vi "CPP-Multiplot.vi"(0 "PlotArray":cluster{dbl[], dbl[]}[](array[cluster]), 1 "Job Directory":path) -> (2 "Saved Automatically?":bool, 3 "gnuplotScript":string, 4 "Plot data file":path)   [LabVIEW 2017]
uses:
  gnuplotScriptComponents/plotstyle.ctl
  gnuplotScriptComponents/graphPeripherals.ctl
  gnuplotScriptComponents/minAndMax.ctl
  gnuplotScriptComponents/AutoManualNumber.ctl
  gnuplotScriptComponents/ticsAndGrids.ctl
  gnuplotScriptComponents/tics.ctl
  gnuplotScriptComponents/grids.ctl
  gnuplotScriptComponents/legendProperties.ctl
  gnuplotScriptComponents/legendAppearance.ctl
  gnuplotScriptComponents/alignment.ctl
  gnuplotScriptComponents/at.ctl
  gnuplotScriptComponents/margins.ctl
  gnuplotScriptComponents/source.ctl
  gnuplotScriptComponents/Master_Legend.ctl
  gnuplotScriptComponents/MasterPeripherals.ctl
  Error bar Type.ctl
  gnuplotScriptComponents/axisName.ctl
  Results_plotter_Global.vi
panel:
  out "Multi_Plot":bool
  in  "OpenLogfile?":bool
  in  "Show Script Editor?":bool
  in  "Tab Control":T1(tab)=enum."Appearance"
  in  "Each Graph contains:":T2=enum."Series"
  in  "Rows from:":T2=enum."Until done"
  in  "Columns from:":T2=enum."Yellow Filter"
  in  "Margins":T3={"Top"=2.0, "Bottom"=2.0, "Left"=2.0, "Right"=2.0}
  in  "Height (in)":dbl=7.0 min=0.5 step=0.5 format="%.1f"
  in  "Width (in)":dbl=10.0 min=0.5 step=0.5 format="%.1f"
  in  "nRows":u8=3 min=1
  in  "nCols":u8=3 min=1
  in  "ScaleAdjust":dbl=0.9 min=0.1 max=2.0 step=0.1
  in  "PlotTitlesNeed $$?":bool=TRUE
  in  "Show Channels with range of Values?":bool
  in  "ManualPlotTitles":string[](array[string])
  out "AutoPlotTitles":string[](array[string])
  in  "Individual Plot Titles":bool=TRUE
  in  "Page Title Pre Block":string
  in  "Page Title Post Block":string
  in  "Values to include in Page Title":i32[](listbox)
  in  "Plot Title Offset (characters)":cluster{"horizontal":dbl, "vertical":dbl}
  out "Final Title":string
  in  "PlotNamesNeed $$?":bool=TRUE
  in  "Plot Legends Manual":string[](array[string])
  in  "Plotstyles":T4[](array[typedef])=[{"Style"="linespoints", "Color"=16711680, "PointType"=1, "PointSize"=1.0, "LineWidth"=1.0, "LineType"=1}, {"Style"="linespoints", "Color"=16860, "PointType"=2, "PointSize"=1.0, "LineWidth"=1.0, "LineType"=1}, {"Style"="linespoints", "Color"=51228, "PointType"=3, "PointSize"=1.0, "LineWidth"=1.0, "LineType"=1}, {"Style"="linespoints", "Color"=0, "PointType"=4, "PointSize"=1.0, "LineWidth"=1.0, "LineType"=1}, {"Style"="linespoints", "Color"=9567230, "PointType"=5, "PointSize"=1.0, "LineWidth"=1.0, "LineType"=1}, {"Style"="linespoints", "Color"=12369084, "PointType"=6, "PointSize"=1.0, "LineWidth"=1.0, "LineType"=1}, {"Style"="linespoints", "Color"=15667967, "PointType"=7, "PointSize"=1.0, "LineWidth"=1.0, "LineType"=1}, {"Style"="linespoints", "Color"=15400704, "PointType"=8, "PointSize"=1.0, "LineWidth"=1.0, "LineType"=1}, {"Style"="linespoints", "Color"=128, "PointType"=9, "PointSize"=1.0, "LineWidth"=1.0, "LineType"=1}, {"Style"="linespoints", "Color"=8404992, "PointType"=10, "PointSize"=1.0, "LineWidth"=1.0, "LineType"=1}, {"Style"="linespoints", "Color"=6737151, "PointType"=11, "PointSize"=1.0, "LineWidth"=1.0, "LineType"=1}, {"Style"="linespoints", "Color"=8388672, "PointType"=12, "PointSize"=1.0, "LineWidth"=1.0, "LineType"=1}, {"Style"="linespoints", "Color"=16740303, "PointType"=13, "PointSize"=1.0, "LineWidth"=1.0, "LineType"=1}, {"Style"="linespoints", "Color"=16764006, "PointType"=14, "PointSize"=1.0, "LineWidth"=1.0, "LineType"=1}, {"Style"="linespoints", "Color"=8421376, "PointType"=15, "PointSize"=1.0, "LineWidth"=1.0, "LineType"=1}, {"Style"="linespoints", "Color"=65408, "PointType"=16, "PointSize"=1.0, "LineWidth"=1.0, "LineType"=1}] caption="Style                              Colour  PointType    PointSize     Linewidth      Linestyle" {"LineType" min=1 max=6 step=1; "LineWidth" min=1 max=6 step=1; "PointSize" min=0 step=0.1}
  out "Plot Legends Auto":string[](array[string])
  out "No of Series supplied":i32
  out "No of Graph Slots Available":i32
  in  "Plot Legends":bool=TRUE
  in  "Error Bar Type":T5
  in  "X axis label":enum32{"Autolabel", "Manual Label"}(tab)
  out "X or theta label":string
  in  "X or theta label Manual":string
  in  "LegendProperties":T6={"Appearance"={"layout"="", "text-sample order"="", "key order"="", "surroundingBox"="", "MaxRows"=0, "MaxCols"=0, "WidthAdjust"=0.0}, "Alignment"={"Horizontal"="", "Vertical"=""}, "Location"="auto", "\"At\" location"={"XcoordSys"="", "YcoordSys"="", "Xvalue"=0.0, "Yvalue"=0.0}}
  in  "Y/R tics And Grids":T10={"tics"={"ticMin"=0.0, "ticStep"=5.0, "ticMax"=0.0, "minorDivsPerMajor"=2, "ticSpacing"=enum."Approx n Tics (rounded)", "ticPosition"=enum."Inside, no mirror"}, "Grids"={"Gridlines"=enum."No grids", "Zeroaxis"=enum."No zero axis"}, "Mapping"=enum."Lin"}
  in  "X/Theta tics And Grids":T10={"tics"={"ticMin"=0.0, "ticStep"=5.0, "ticMax"=0.0, "minorDivsPerMajor"=2, "ticSpacing"=enum."Approx n Tics (rounded)", "ticPosition"=enum."Inside, no mirror"}, "Grids"={"Gridlines"=enum."Major grid", "Zeroaxis"=enum."No zero axis"}, "Mapping"=enum."Lin"}
  in  "PlotType":enum32{"XY", "Polar", "Time"}(tab)
  in  "yAxisBounds":T13={"Min"={"Auto"=TRUE, "Value"=0.0}, "Max"={"Auto"=TRUE, "Value"=0.0}}
  in  "Additional XYgnuplot":string
  in  "xAxisBounds":T13={"Min"={"Auto"=TRUE, "Value"=0.0}, "Max"={"Auto"=TRUE, "Value"=0.0}}
  in  "Set bounds using XY Plot \non Results file plotter":bool
  in  "Angle Units":bool=TRUE
  in  "AngleMode":string(combo)="Compass"
  in  "wrapGapsUpTo:":dbl=30.0 step=0.1
  in  "Additional Polar gnuplot":string
  in  "rAxisBounds":T13={"Min"={"Auto"=FALSE, "Value"=0.0}, "Max"={"Auto"=FALSE, "Value"=1.5}}
  out "Time format?":bool
  in  "Time/Date Format":string(combo)="%I:%M %p\\n%d-%b-%y"
  in  "Select Time Zone":u32(ring)=142 items=["Abbreviation (Time Zone Name)", "A (Alpha Time Zone)", "ACDT (Australian Central Daylight Time  CDT ‚Äì Central Daylight Time CDST ‚Äì Central Daylight Savings Time)", "ACST (Australian Central Standard Time  CST ‚Äì Central Standard Time)", "ACT (Acre Time)", "ACT (Australian Central Time)", "ACWST (Australian Central Western Standard Time)", "ADT (Arabia Daylight Time  AST ‚Äì Arabia Summer Time)", "ADT (Atlantic Daylight Time  ADST ‚Äì Atlantic Daylight Saving Time AST ‚Äì Atlantic Summer Time  HAA ‚Äì Heure Avancv©e de l'Atlantique (French))", "AEDT (Australian Eastern Daylight Time  EDT ‚Äì Eastern Daylight Time EDST ‚Äì Eastern Daylight Saving Time)", "AEST (Australian Eastern Standard Time  EST ‚Äì Eastern Standard Time AET ‚Äì Australian Eastern Time)", "AET (Australian Eastern Time)", "AFT (Afghanistan Time)", "AKDT (Alaska Daylight Time  ADST ‚Äì Alaska Daylight Saving Time)", "AKST (Alaska Standard Time  AT ‚Äì Alaska Time)", "ALMT (Alma-Ata Time)", "AMST (Amazon Summer Time)", "AMST (Armenia Summer Time  AMDT ‚Äì Armenia Daylight Time)", "AMT (Amazon Time)", "AMT (Armenia Time)", "ANAST (Anadyr Summer Time)", "ANAT (Anadyr Time)", "AQTT (Aqtobe Time)", "ART (Argentina Time)", "AST (Arabia Standard Time  AST ‚Äì Arabic Standard Time AST ‚Äì Al Manamah Standard Time)", "AST (Atlantic Standard Time  AT ‚Äì Atlantic Time  AST ‚Äì Tiempo Estv°ndar del Atlv°ntico (Spanish) HNA ‚Äì Heure Normale de l'Atlantique (French))", "AT (Atlantic Time)", "AWDT (Australian Western Daylight Time  WDT ‚Äì Western Daylight Time WST ‚Äì Western Summer Time)", "AWST (Australian Western Standard Time  WST ‚Äì Western Standard Time WAT ‚Äì Western Australia Time)", "AZOST (Azores Summer Time  AZODT ‚Äì Azores Daylight Time)", "AZOT (Azores Time  AZOST ‚Äì Azores Standard Time)", "AZST (Azerbaijan Summer Time)", "AZT (Azerbaijan Time)", "AoE (Anywhere on Earth)", "B (Bravo Time Zone)", "BNT (Brunei Darussalam Time  BDT ‚Äì Brunei Time)", "BOT (Bolivia Time)", "BRST (Brasv?lia Summer Time  BST ‚Äì Brazil Summer Time BST ‚Äì Brazilian Summer Time)", "BRT (Brasv?lia Time  BT ‚Äì Brazil Time BT ‚Äì Brazilian Time)", "BST (Bangladesh Standard Time)", "BST (Bougainville Standard Time)", "BST (British Summer Time  BDT ‚Äì British Daylight Time BDST ‚Äì British Daylight Saving Time)", "BTT (Bhutan Time)", "C (Charlie Time Zone)", "CAST (Casey Time)", "CAT (Central Africa Time)", "CCT (Cocos Islands Time)", "CDT (Central Daylight Time  CDST ‚Äì Central Daylight Saving Time NACDT ‚Äì North American Central Daylight Time  HAC ‚Äì Heure Avancv©e du Centre (French))", "CDT (Cuba Daylight Time)", "CEST (Central European Summer Time  CEDT ‚Äì Central European Daylight Time ECST ‚Äì European Central Summer Time  MESZ ‚Äì Mitteleuropv§ische Sommerzeit (German))", "CET (Central European Time  ECT ‚Äì European Central Time CET ‚Äì Central Europe Time  MEZ ‚Äì Mitteleuropv§ische Zeit (German))", "CHADT (Chatham Island Daylight Time  CDT ‚Äì Chatham Daylight Time)", "CHAST (Chatham Island Standard Time)", "CHOST (Choibalsan Summer Time  CHODT ‚Äì Choibalsan Daylight Time CHODST ‚Äì Choibalsan Daylight Saving Time)", "CHOST (Choibalsan Summer Time)", "CHOT (Choibalsan Time)", "CHUT (Chuuk Time)", "CIDST (Cayman Islands Daylight Saving Time)", "CIST (Cayman Islands Standard Time  CIT ‚Äì Cayman Islands Time)", "CKT (Cook Island Time)", "CLST (Chile Summer Time  CLDT ‚Äì Chile Daylight Time)", "CLT (Chile Standard Time  CT ‚Äì Chile Time CLST ‚Äì Chile Standard Time)", "COT (Colombia Time)", "CST (Central Standard Time  CT ‚Äì Central Time NACST ‚Äì North American Central Standard Time  CST ‚Äì Tiempo Central Estv°ndar (Spanish) HNC ‚Äì Heure Normale du Centre (French))", "CST (China Standard Time)", "CST (Cuba Standard Time)", "CT (Central Time)", "CVT (Cape Verde Time)", "CXT (Christmas Island Time)", "ChST (Chamorro Standard Time  GST ‚Äì Guam Standard Time)", "D (Delta Time Zone)", "DAVT (Davis Time)", "DDUT (Dumont-d'Urville Time)", "E (Echo Time Zone)", "EASST (Easter Island Summer Time  EADT ‚Äì Easter Island Daylight Time)", "EAST (Easter Island Standard Time)", "EAT (Eastern Africa Time  EAT ‚Äì East Africa Time)", "ECT (Ecuador Time)", "EDT (Eastern Daylight Time  EDST ‚Äì Eastern Daylight Savings Time NAEDT ‚Äì North American Eastern Daylight Time  HAE ‚Äì Heure Avancv©e de l'Est (French) EDT ‚Äì Tiempo de verano del Este (Spanish))", "EEST (Eastern European Summer Time  EEDT ‚Äì Eastern European Daylight Time  OESZ ‚Äì Osteuropv§ische Sommerzeit (German))", "EET (Eastern European Time  OEZ ‚Äì Osteuropv§ische Zeit (German))", "EGST (Eastern Greenland Summer Time  EGST ‚Äì East Greenland Summer Time)", "EGT (East Greenland Time  EGT ‚Äì Eastern Greenland Time)", "EST (Eastern Standard Time  ET ‚Äì Eastern Time  NAEST ‚Äì North American Eastern Standard Time  ET ‚Äì Tiempo del Este (Spanish) HNE ‚Äì Heure Normale de l'Est (French))", "ET (Eastern Time)", "F (Foxtrot Time Zone)", "FET (Further-Eastern European Time)", "FJST (Fiji Summer Time  FJDT ‚Äì Fiji Daylight Time)", "FJT (Fiji Time)", "FKST (Falkland Islands Summer Time  FKDT ‚Äì Falkland Island Daylight Time)", "FKT (Falkland Island Time  FKST ‚Äì Falkland Island Standard Time)", "FNT (Fernando de Noronha Time)", "G (Golf Time Zone)", "GALT (Galapagos Time)", "GAMT (Gambier Time  GAMT ‚Äì Gambier Islands Time)", "GET (Georgia Standard Time)", "GFT (French Guiana Time)", "GILT (Gilbert Island Time)", "GMT (Greenwich Mean Time  \"‚Äì Coordinated Universal Time GT ‚Äì Greenwich Time)", "GST (Gulf Standard Time)", "GST (South Georgia Time)", "GYT (Guyana Time)", "H (Hotel Time Zone)", "HADT (Hawaii-Aleutian Daylight Time  HDT ‚Äì Hawaii Daylight Time)", "HAST (Hawaii-Aleutian Standard Time  HST ‚Äì Hawaii Standard Time)", "HKT (Hong Kong Time)", "HOVST (Hovd Summer Time  HOVDT ‚Äì Hovd Daylight Time HOVDST ‚Äì Hovd Daylight Saving Time)", "HOVST (Hovd Summer Time)", "HOVT (Hovd Time)", "I (India Time Zone)", "ICT (Indochina Time)", "IDT (Israel Daylight Time)", "IOT (Indian Chagos Time)", "IRDT (Iran Daylight Time  IRST ‚Äì Iran Summer Time IDT ‚Äì Iran Daylight Time)", "IRKST (Irkutsk Summer Time)", "IRKT (Irkutsk Time)", "IRST (Iran Standard Time  IT ‚Äì Iran Time)", "IST (India Standard Time  IT ‚Äì India Time IST ‚Äì Indian Standard Time)", "IST (Irish Standard Time  IST ‚Äì Irish Summer Time)", "IST (Israel Standard Time)", "JST (Japan Standard Time)", "K (Kilo Time Zone)", "KGT (Kyrgyzstan Time)", "KOST (Kosrae Time)", "KRAST (Krasnoyarsk Summer Time)", "KRAT (Krasnoyarsk Time)", "KST (Korea Standard Time  KST ‚Äì Korean Standard Time KT ‚Äì Korea Time)", "KUYT (Kuybyshev Time  SAMST ‚Äì Samara Summer Time)", "L (Lima Time Zone)", "LHDT (Lord Howe Daylight Time)", "LHST (Lord Howe Standard Time)", "LINT (Line Islands Time)", "M (Mike Time Zone)", "MAGST (Magadan Summer Time  MAGST ‚Äì Magadan Island Summer Time)", "MAGT (Magadan Time  MAGT ‚Äì Magadan Island Time)", "MART (Marquesas Time)", "MAWT (Mawson Time)", "MDT (Mountain Daylight Time  MDST ‚Äì Mountain Daylight Saving Time NAMDT ‚Äì North American Mountain Daylight Time  HAR ‚Äì Heure Avancv©e des Rocheuses (French))", "MHT (Marshall Islands Time)", "MMT (Myanmar Time)", "MSD (Moscow Daylight Time  Moscow Summer Time)", "MSK (Moscow Standard Time  MCK ‚Äì Moscow Time)", "MST (Mountain Standard Time  MT ‚Äì Mountain Time NAMST ‚Äì North American Mountain Standard Time  HNR ‚Äì Heure Normale des Rocheuses (French))", "MT (Mountain Time)", "MUT (Mauritius Time)", "MVT (Maldives Time)", "MYT (Malaysia Time  MST ‚Äì Malaysian Standard Time)", "N (November Time Zone)", "NCT (New Caledonia Time)", "NDT (Newfoundland Daylight Time  HAT ‚Äì Heure Avancv©e de Terre-Neuve (French))", "NFT (Norfolk Time  NFT ‚Äì Norfolk Island Time)", "NOVST (Novosibirsk Summer Time  OMSST ‚Äì Omsk Summer Time)", "NOVT (Novosibirsk Time  OMST ‚Äì Omsk Standard Time)", "NPT (Nepal Time)", "NRT (Nauru Time)", "NST (Newfoundland Standard Time  HNT ‚Äì Heure Normale de Terre-Neuve (French))", "NUT (Niue Time)", "NZDT (New Zealand Daylight Time)", "NZST (New Zealand Standard Time)", "O (Oscar Time Zone)", "OMSST (Omsk Summer Time  NOVST ‚Äì Novosibirsk Summer Time)", "OMST (Omsk Standard Time  OMST ‚Äì Omsk Time NOVT ‚Äì Novosibirsk Time)", "ORAT (Oral Time)", "P (Papa Time Zone)", "PDT (Pacific Daylight Time  PDST ‚Äì Pacific Daylight Saving Time NAPDT ‚Äì North American Pacific Daylight Time  HAP ‚Äì Heure Avancv©e du Pacifique (French))", "PET (Peru Time)", "PETST (Kamchatka Summer Time)", "PETT (Kamchatka Time  PETT ‚Äì Petropavlovsk-Kamchatski Time)", "PGT (Papua New Guinea Time)", "PHOT (Phoenix Island Time)", "PHT (Philippine Time  PST ‚Äì Philippine Standard Time)", "PKT (Pakistan Standard Time  PKT ‚Äì Pakistan Time)", "PMDT (Pierre & Miquelon Daylight Time)", "PMST (Pierre & Miquelon Standard Time)", "PONT (Pohnpei Standard Time)", "PST (Pacific Standard Time  PT ‚Äì Pacific Time NAPST ‚Äì North American Pacific Standard Time  PT ‚Äì Tiempo del Pacv?fico (Spanish) HNP ‚Äì Heure Normale du Pacifique (French))", "PST (Pitcairn Standard Time)", "PT (Pacific Time)", "PWT (Palau Time)", "PYST (Paraguay Summer Time)", "PYT (Paraguay Time)", "PYT (Pyongyang Time  PYST ‚Äì Pyongyang Standard Time)", "PYT (Pyongyang Time)", "Q (Quebec Time Zone)", "QYZT (Qyzylorda Time)", "R (Romeo Time Zone)", "RET (Reunion Time)", "ROTT (Rothera Time)", "S (Sierra Time Zone)", "SAKT (Sakhalin Time)", "SAMT (Samara Time  SAMT ‚Äì Samara Standard Time)", "SAST (South Africa Standard Time  SAST ‚Äì South African Standard Time)", "SBT (Solomon Islands Time  SBT ‚Äì Solomon Island Time)", "SCT (Seychelles Time)", "SGT (Singapore Time  SST ‚Äì Singapore Standard Time)", "SRET (Srednekolymsk Time)", "SRT (Suriname Time)", "SST (Samoa Standard Time)", "SYOT (Syowa Time)", "T (Tango Time Zone)", "TAHT (Tahiti Time)", "TFT (French Southern and Antarctic Time  KIT ‚Äì Kerguelen (Islands) Time)", "TJT (Tajikistan Time)", "TKT (Tokelau Time)", "TLT (East Timor Time)", "TMT (Turkmenistan Time)", "TOT (Tonga Time)", "TVT (Tuvalu Time)", "U (Uniform Time Zone)", "ULAST (Ulaanbaatar Summer Time  ULAST ‚Äì Ulan Bator Summer Time)", "ULAST (Ulaanbaatar Summer Time)", "ULAT (Ulaanbaatar Time  ULAT ‚Äì Ulan Bator Time)", "ULAT (Ulaanbaatar Time)", "UTC (Coordinated Universal Time)", "UYST (Uruguay Summer Time)", "UYT (Uruguay Time)", "UZT (Uzbekistan Time)", "V (Victor Time Zone)", "VET (Venezuelan Standard Time  HLV ‚Äì Hora Legal de Venezuela (Spanish))", "VLAST (Vladivostok Summer Time)", "VLAT (Vladivostok Time)", "VOST (Vostok Time)", "VUT (Vanuatu Time  EFATE ‚Äì Efate Time)", "W (Whiskey Time Zone)", "WAKT (Wake Time)", "WARST (Western Argentine Summer Time)", "WAST (West Africa Summer Time)", "WAT (West Africa Time)", "WEST (Western European Summer Time  WEDT ‚Äì Western European Daylight Time  WESZ ‚Äì Westeuropv§ische Sommerzeit (German))", "WET (Western European Time  GMT ‚Äì Greenwich Mean Time  WEZ ‚Äì Westeuropv§ische Zeit (German))", "WFT (Wallis and Futuna Time)", "WGST (Western Greenland Summer Time  WGST ‚Äì West Greenland Summer Time)", "WGT (West Greenland Time  WGT ‚Äì Western Greenland Time)", "WIB (Western Indonesian Time  WIB ‚Äì Waktu Indonesia Barat)", "WIT (Eastern Indonesian Time  WIT ‚Äì Waktu Indonesia Timur)", "WITA (Central Indonesian Time  WITA ‚Äì Waktu Indonesia Tengah)", "WST (West Samoa Time  ST ‚Äì Samoa Time)", "WST (Western Sahara Summer Time)", "WT (Western Sahara Standard Time  WT ‚Äì Western Sahara Time)", "X (X-ray Time Zone)", "Y (Yankee Time Zone)", "YAKST (Yakutsk Summer Time)", "YAKT (Yakutsk Time)", "YAPT (Yap Time)", "YEKST (Yekaterinburg Summer Time)", "YEKT (Yekaterinburg Time)", "Z (Zulu Time Zone)"]
  out "Time Format String":string="%I:%M %p\\n%d-%b-%y"
  out "Formatted date/time string":string="05:00 PM\\n21-Jan-16"
  out "TZ Shift (hrs)":string="UTC-7.00"
  in  "Y axis label":enum32{"Autolabel", "Manual Label"}(tab)
  out "Y or R label":string
  in  "Y or R label Manual 2":string
  in  "PeripheralsMasterControl":T15=enum."Edges Only"
  in  "Legend Options":T16=enum."Single Legend Below table"
  in  "GraphPeripherals":T17[][](array[typedef])
  out "PlotCommand":string
  in  "Filename Max length":i32=55
  out "File Path Control":path
  out "AuditTrail":string[](array[string])
  out "Desired Legends":string[][](array[string])
  out "original name had conflict":bool
  out "crossplatform problem":bool
  # "Rows/ Columns/ Series from: controls not wired- just a thought for explicit control of what goes where...?"
  # "Overall Page Title"
  # "There are as many graphs as there are titles (from Selector 2)...."
  # "Plot Styles"
  # "Each graph contains plots from Selector 1..."
  # "X/theta"
  # "Y/r"
  # "Shows the numbered line colours and point styles available- well it would, if it didn't disappear every time I update from the repository..!"
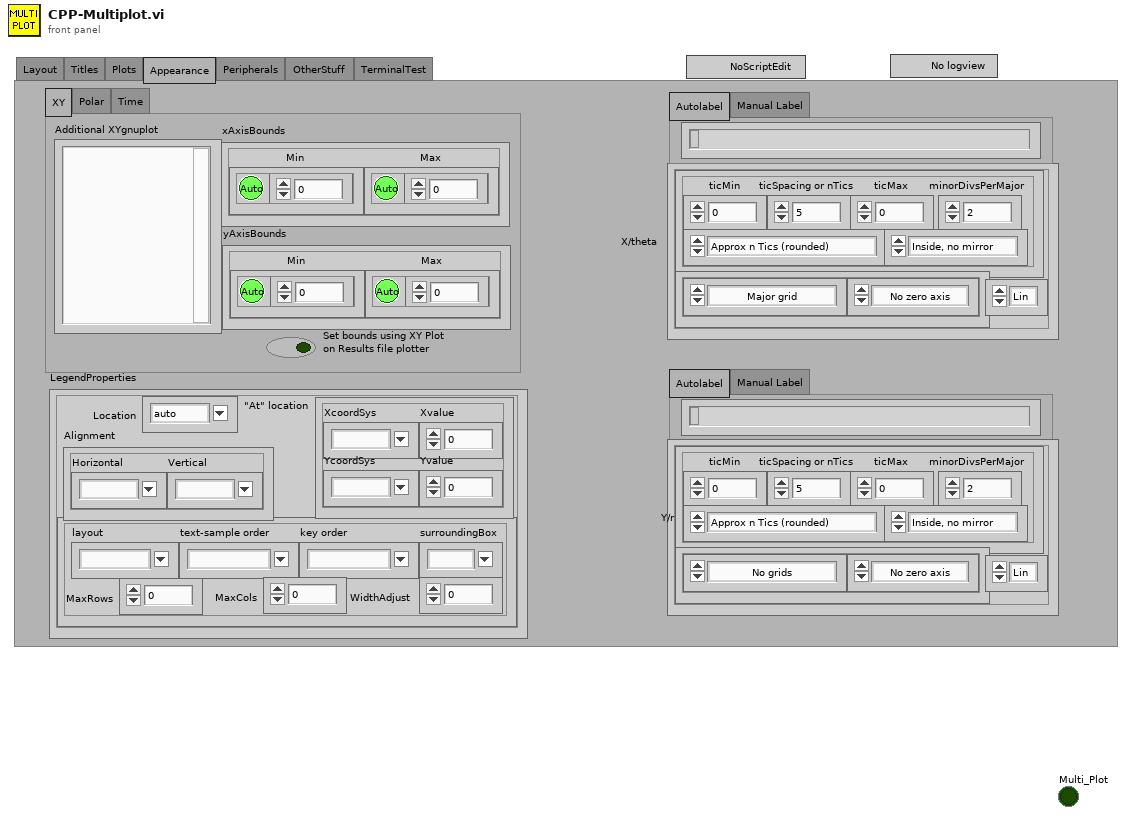
[diagram p1: front panel]
types:
  T1 = enum32{"Layout", "Titles", "Plots", "Appearance", "Peripherals", "OtherStuff ", "TerminalTest"}
  T2 = typedef "source.ctl" = enum16{"Specified:", "Yellow Filter", "Red Filter", "Until done", "Series"}
  T3 = typedef "margins.ctl" = cluster{"Top":dbl, "Bottom":dbl, "Left":dbl, "Right":dbl}
  T4 = typedef "plotstyle.ctl" = cluster{"Style":string, "Color":u32, "PointType":i32, "PointSize":sgl, "LineWidth":sgl, "LineType":u8}
  T5 = typedef "Error bar Type.ctl" = enum16{"Standard Error", "Separate upper and lower"}
  T6 = typedef "legendProperties.ctl" = cluster{"Appearance":T7, "Alignment":T8, "Location":string, "\"At\" location":T9}
  T7 = typedef "legendAppearance.ctl" = cluster{"layout":string, "text-sample order":string, "key order":string, "surroundingBox":string, "MaxRows":u32, "MaxCols":u32, "WidthAdjust":dbl}
  T8 = typedef "alignment.ctl" = cluster{"Horizontal":string, "Vertical":string}
  T9 = typedef "at.ctl" = cluster{"XcoordSys":string, "YcoordSys":string, "Xvalue":dbl, "Yvalue":dbl}
  T10 = typedef "ticsAndGrids.ctl" = cluster{"tics":T11, "Grids":T12, "Mapping":enum8{"Lin", "Log"}}
  T11 = typedef "tics.ctl" = cluster{"ticMin":dbl, "ticStep":dbl, "ticMax":dbl, "minorDivsPerMajor":i32, "ticSpacing":enum16{"Auto Tics", "Fixed spacing", "Fixed Minimum and Spacing", "Start, Spacing and Maximum", "Approx n Tics (rounded)"}, "ticPosition":enum16{"Inside, no mirror", "Inside, mirrored", "Outside, no mirror", "Outside, mirrored", "Invisible"}}
  T12 = typedef "grids.ctl" = cluster{"Gridlines":enum16{"No grids", "Major grid", "Minor grid", "Major and Minor"}, "Zeroaxis":enum16{"No zero axis", "Show zero axis"}}
  T13 = typedef "minAndMax.ctl" = cluster{"Min":T14, "Max":T14}
  T14 = typedef "AutoManualNumber.ctl" = cluster{"Auto":bool, "Value":dbl}
  T15 = typedef "MasterPeripherals.ctl" = enum16{"Use Table", "Titles On", "Edges Only", "All Off"}
  T16 = typedef "Master_Legend.ctl" = enum16{"No Legend", "Single Legend Below table", "Legend as per array"}
  T17 = typedef "graphPeripherals.ctl" = cluster{"title":bool, "key":bool, "Xtic":bool, "Ytic":bool, "Xlab":bool, "Ylab":bool}
  T18 = typedef "Error_bars.ctl" = cluster{"Upper":string[], "Lower":string[], "St Error":string[]}
  T19 = typedef "axisName.ctl" = string
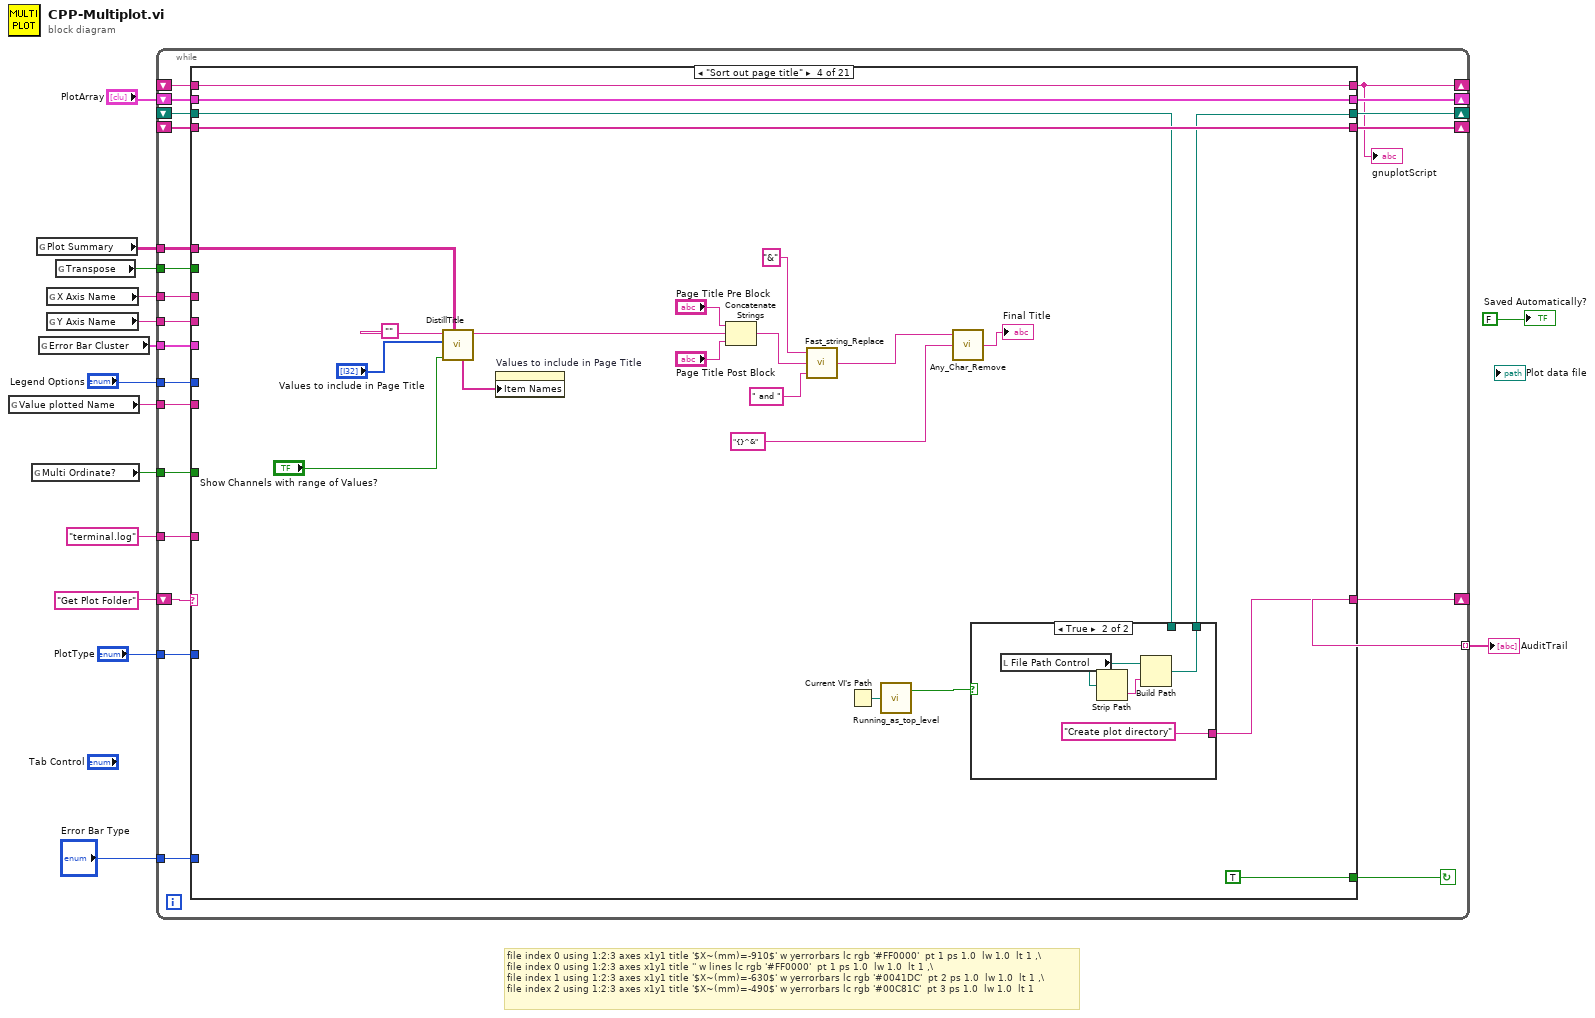
[diagram p0: block diagram]
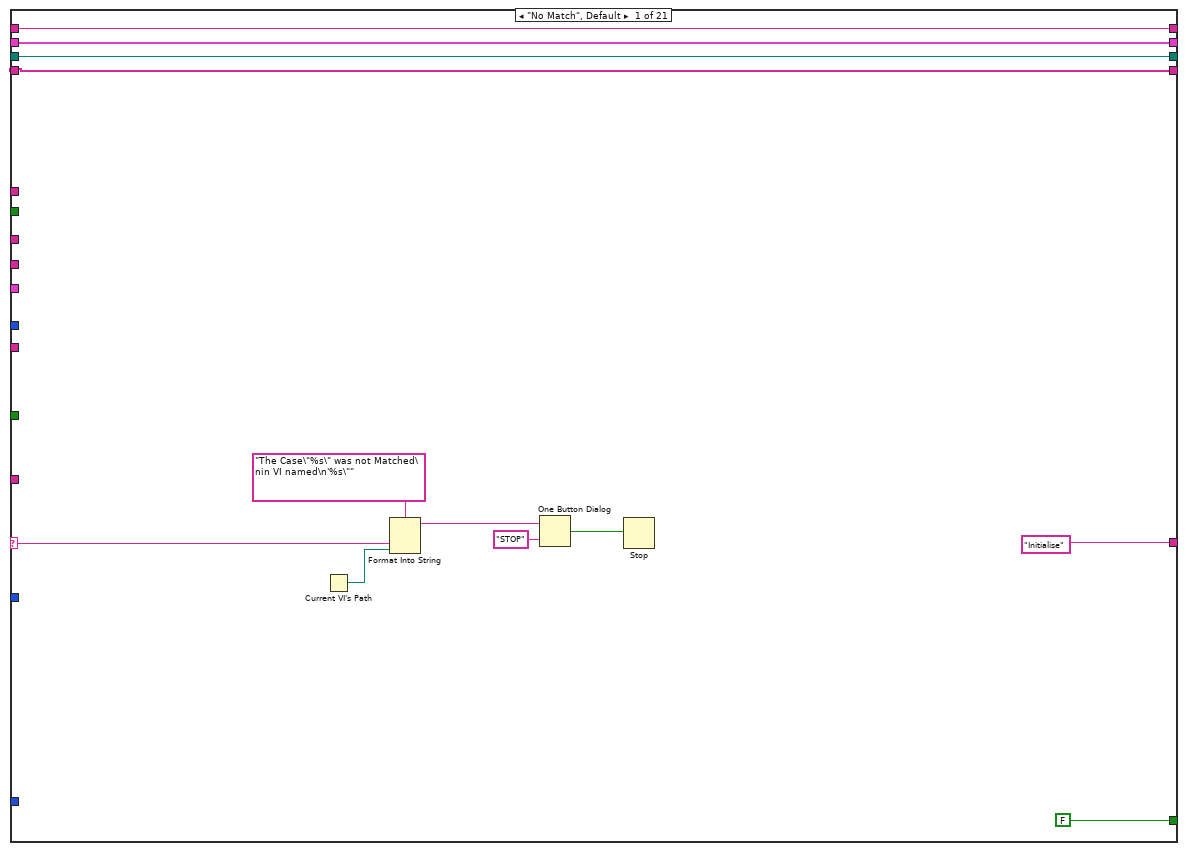
[diagram p2: hidden frame]
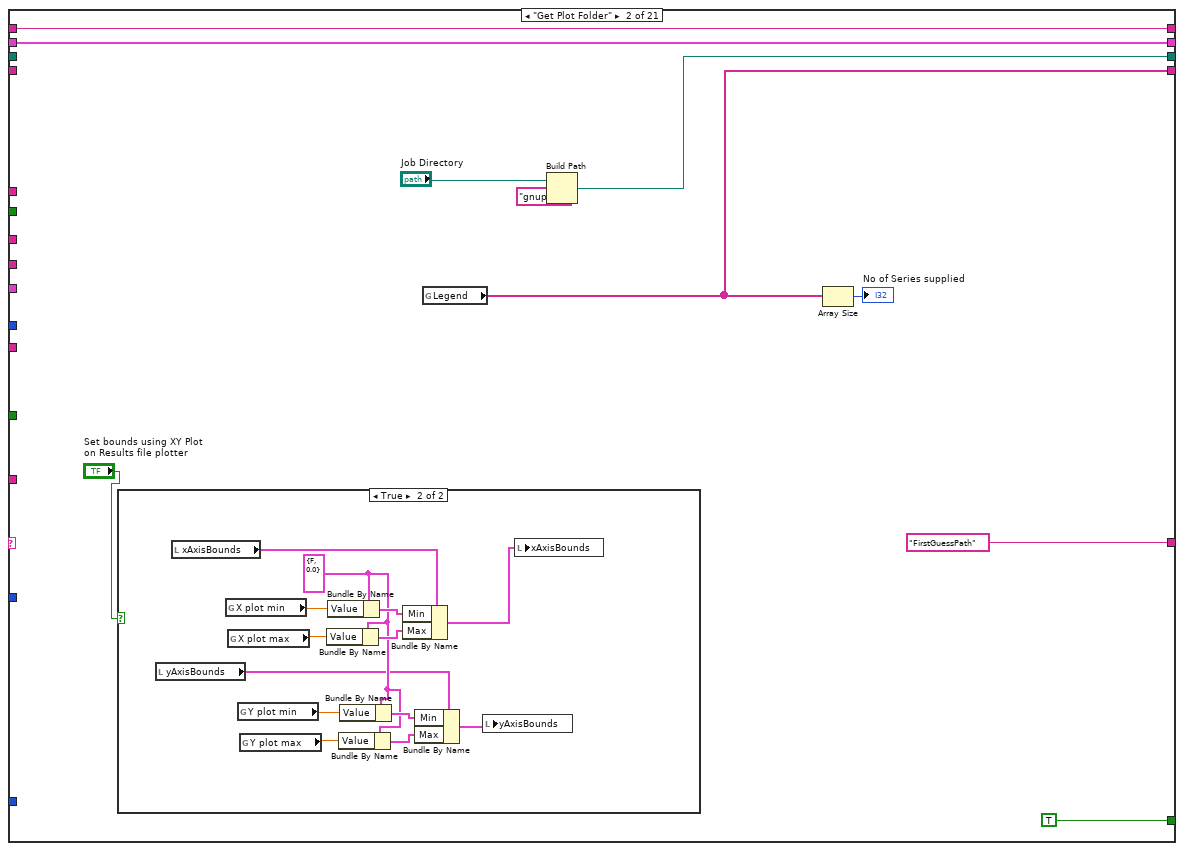
[diagram p3: hidden frame]
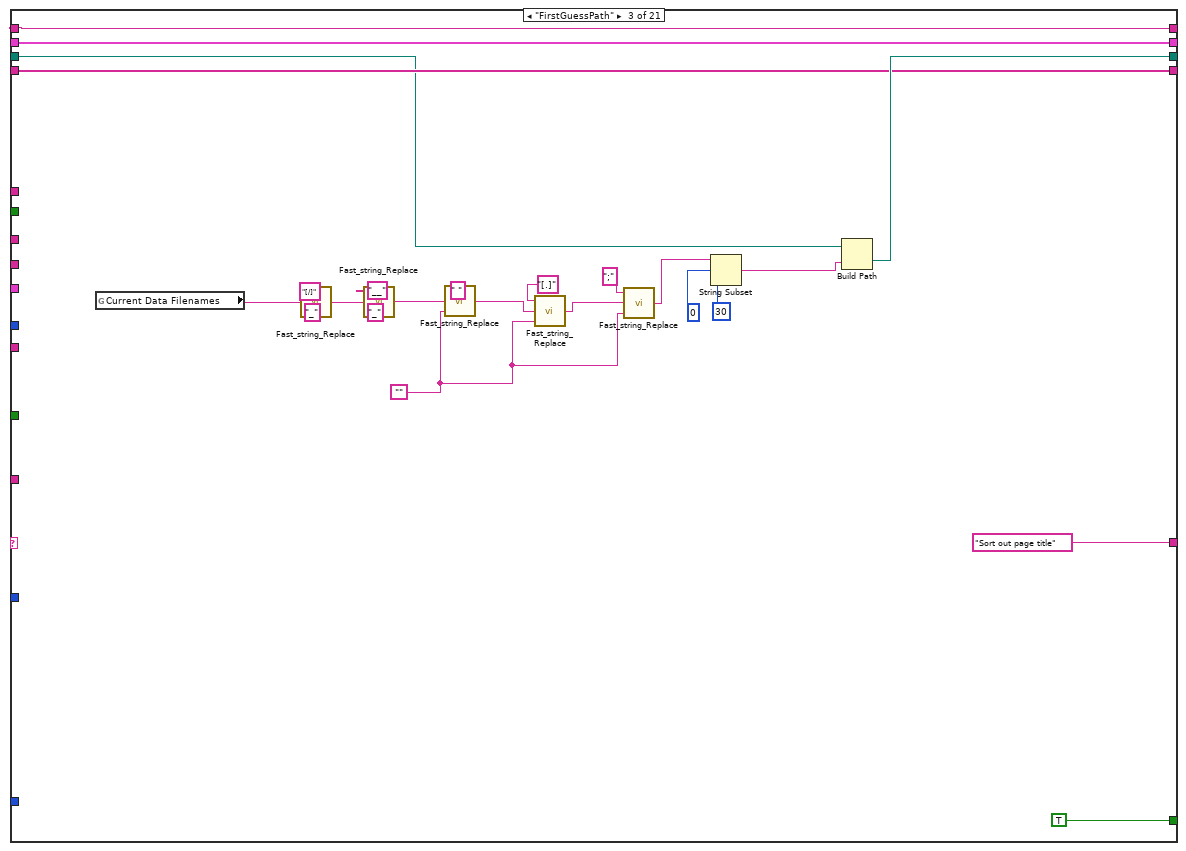
[diagram p5: hidden frame]
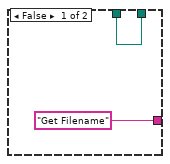
[diagram p6: hidden frame]
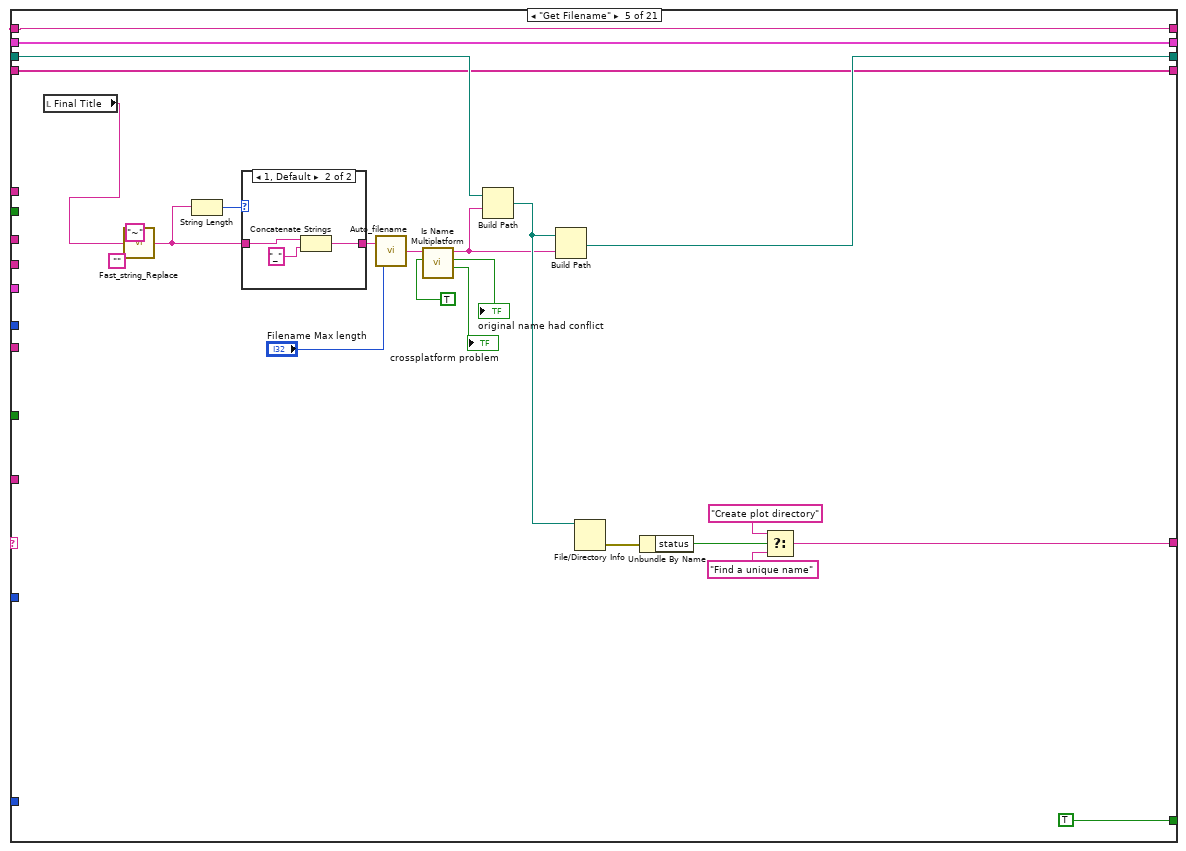
[diagram p7: hidden frame]
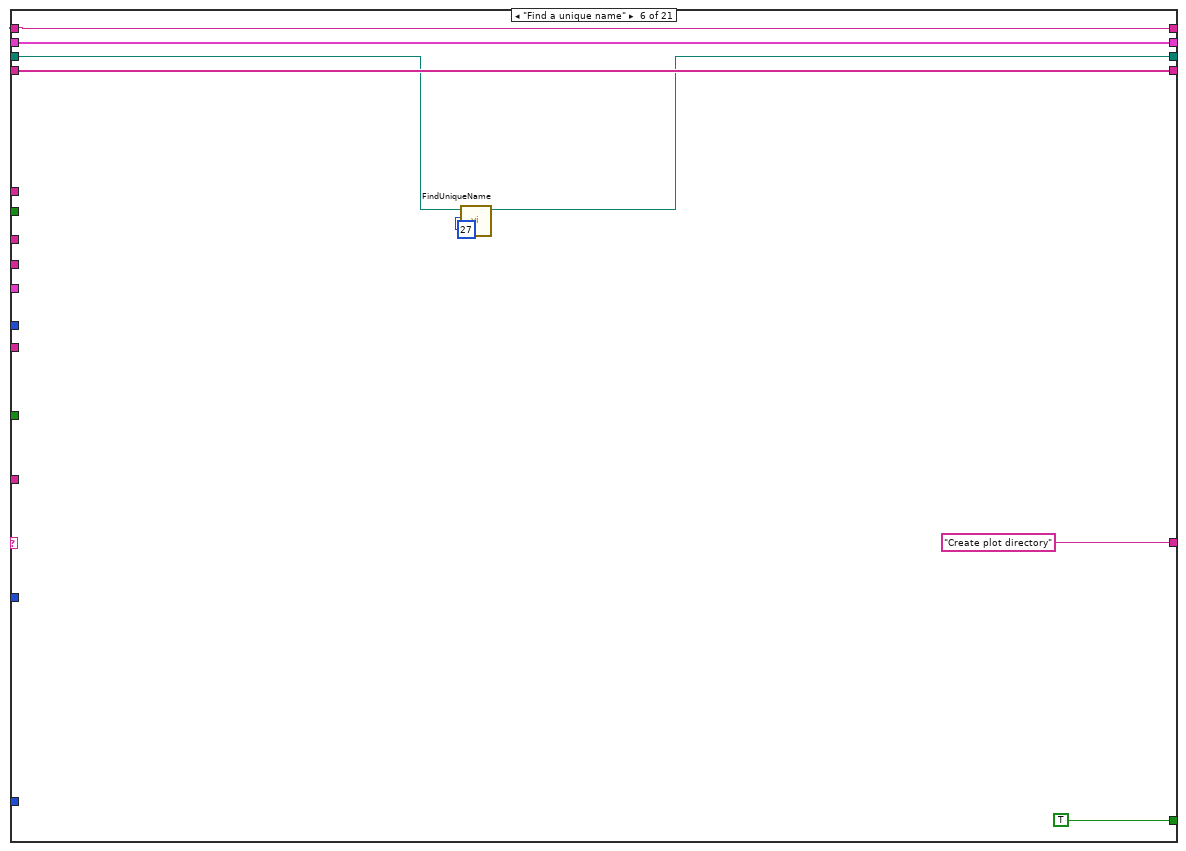
[diagram p9: hidden frame]
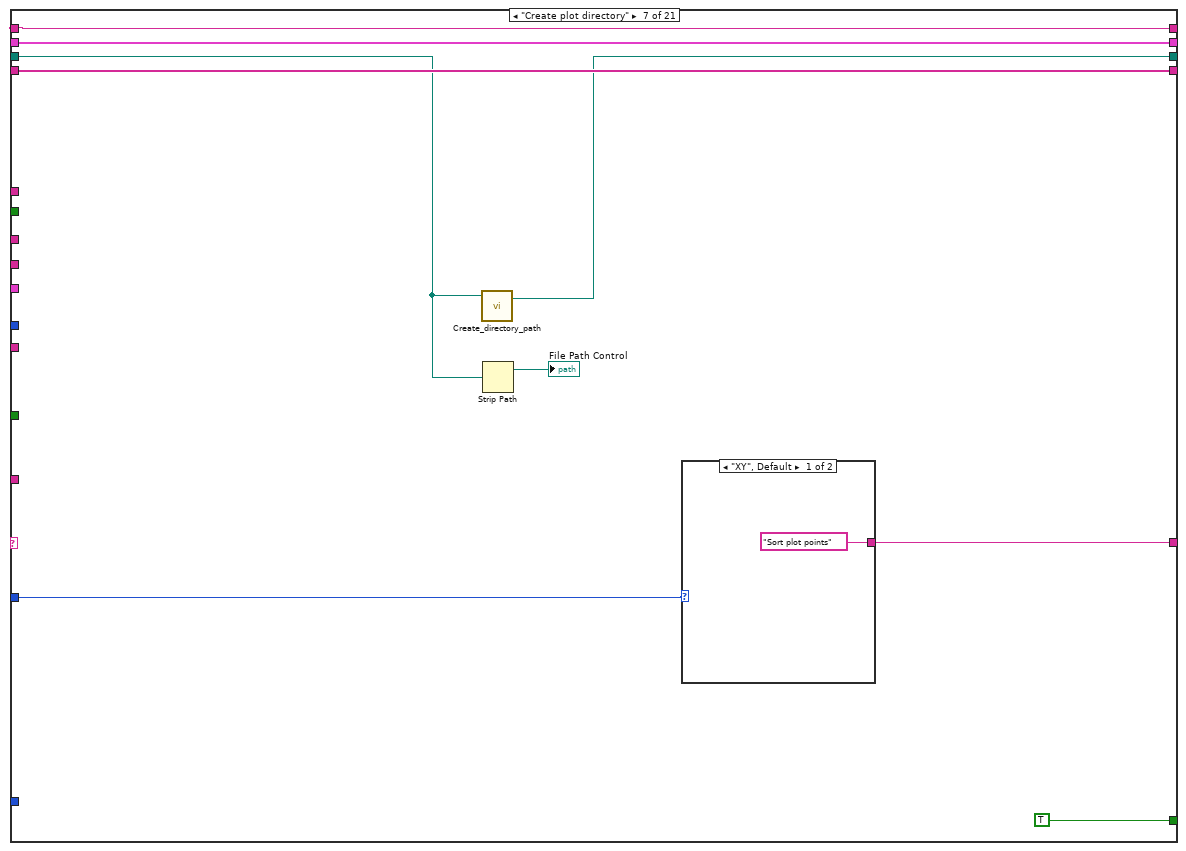
[diagram p10: hidden frame]
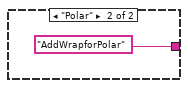
[diagram p11: hidden frame]
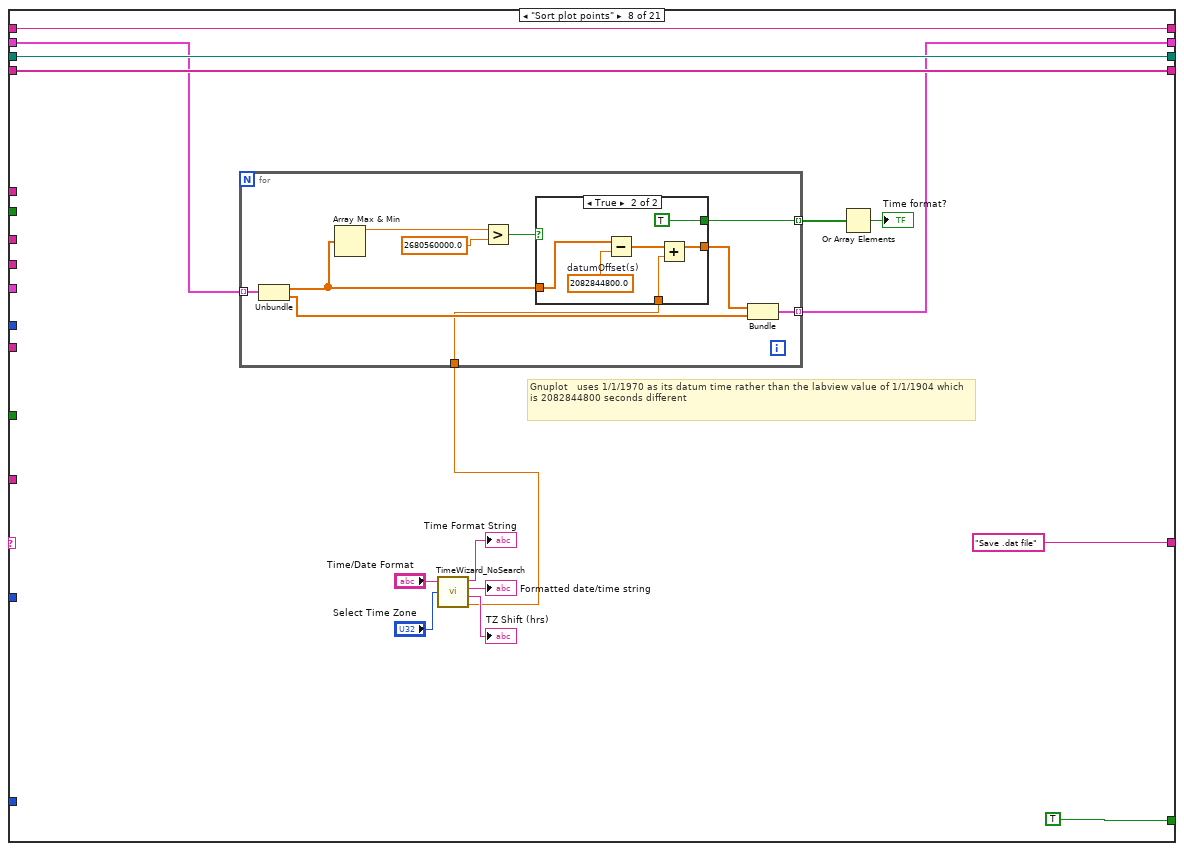
[diagram p12: hidden frame]
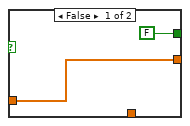
[diagram p13: hidden frame]
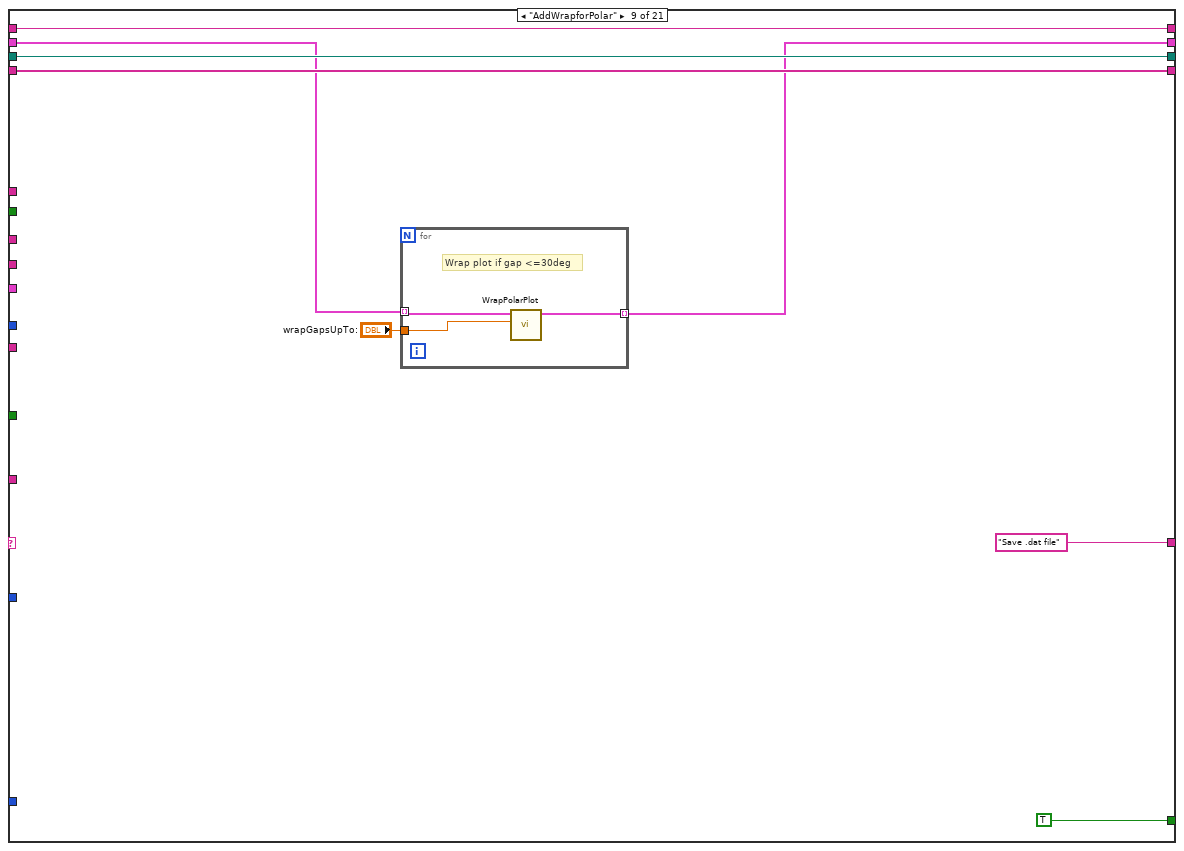
[diagram p14: hidden frame]
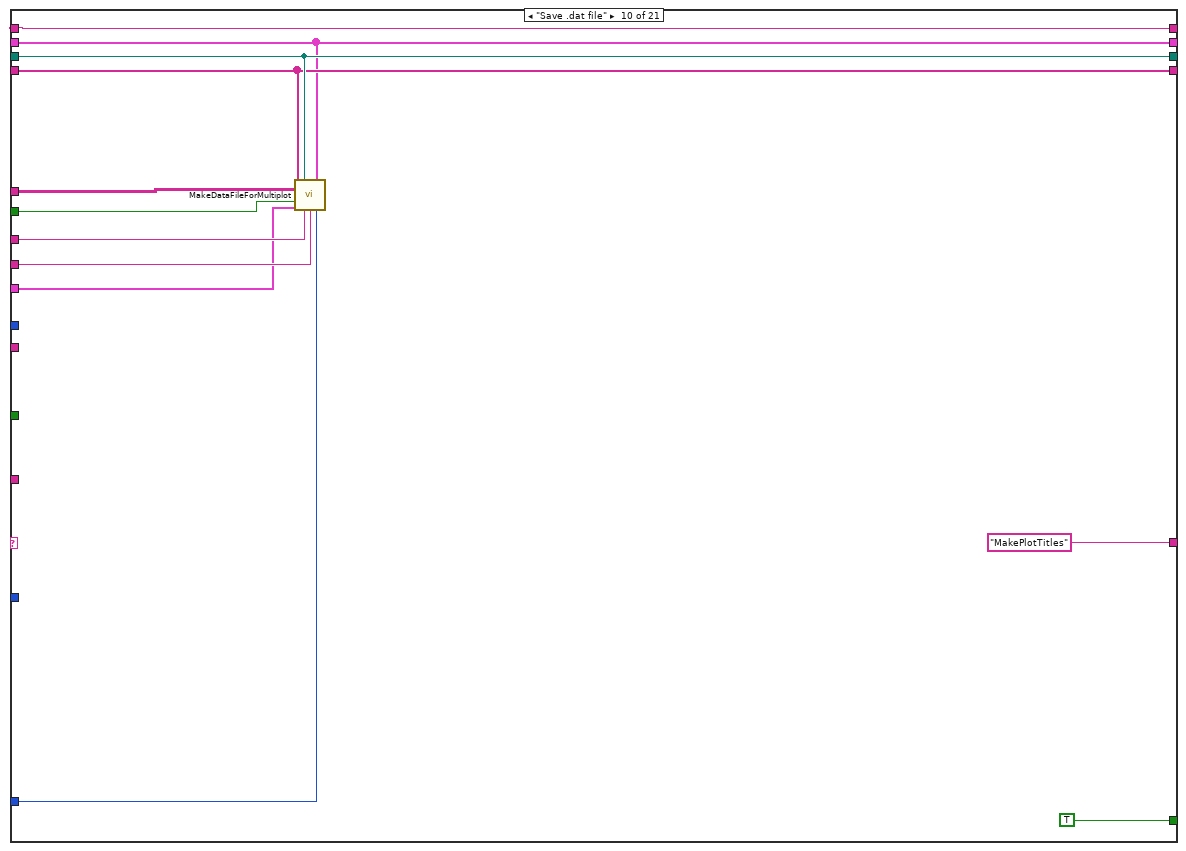
[diagram p15: hidden frame]
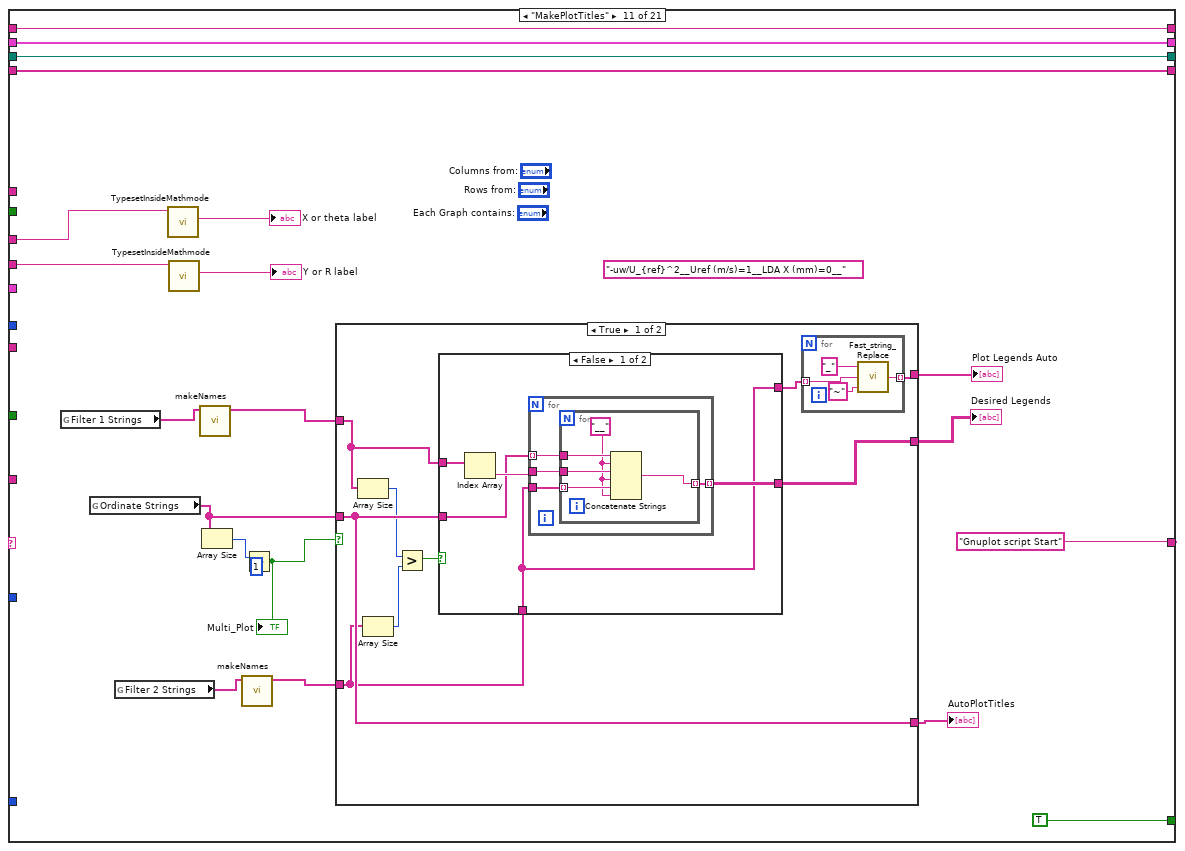
[diagram p16: hidden frame]
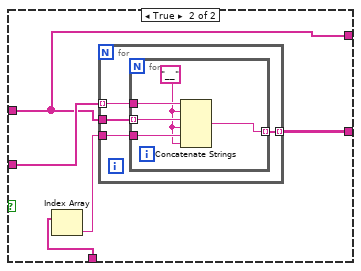
[diagram p17: hidden frame]
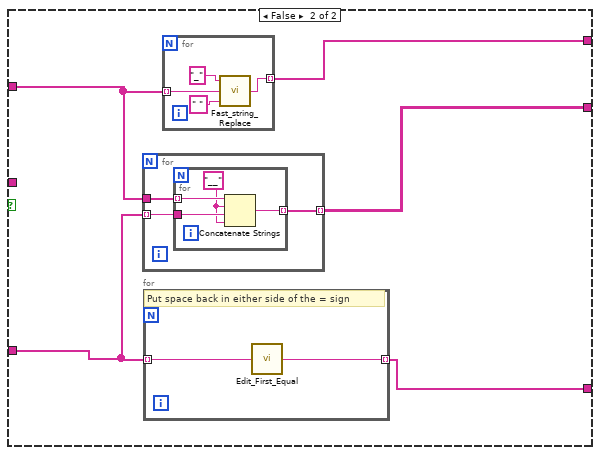
[diagram p18: hidden frame]
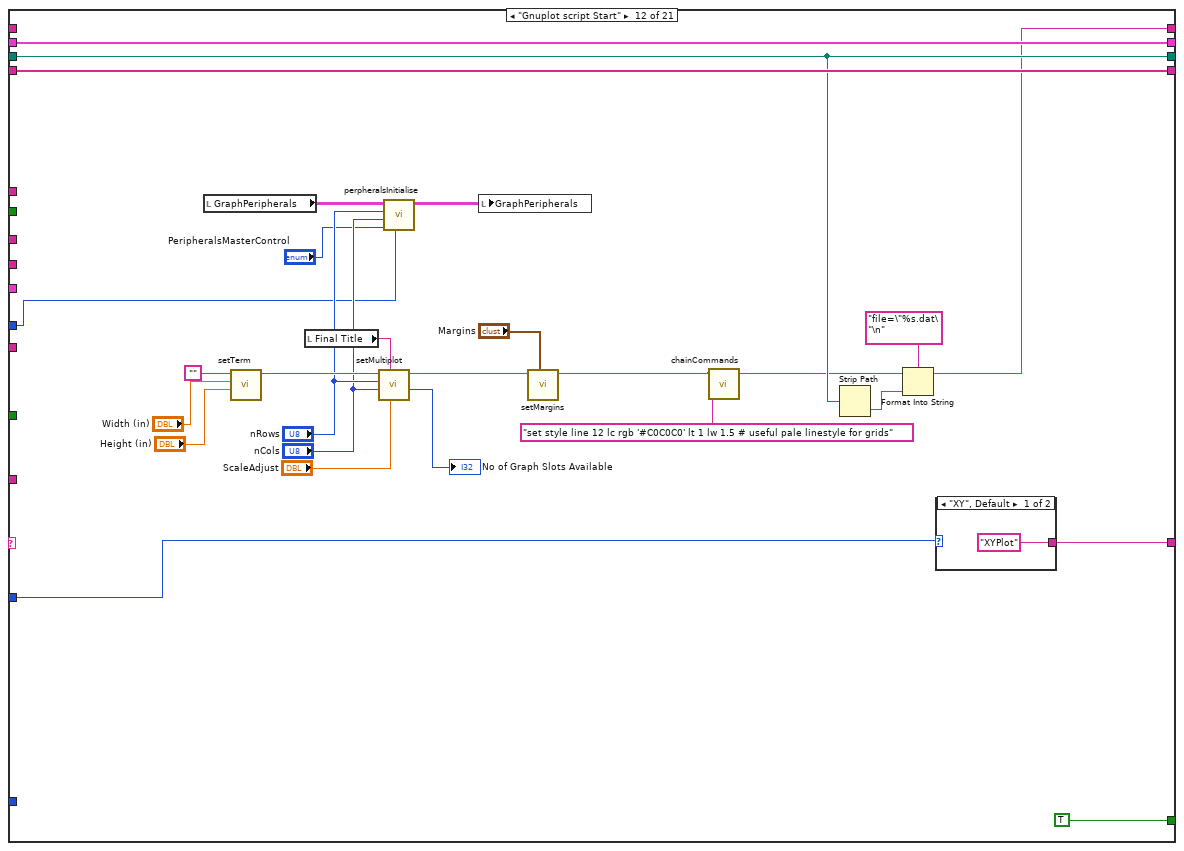
[diagram p19: hidden frame]
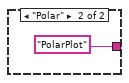
[diagram p20: hidden frame]
diagram:
  # "file index 0 using 1:2:3 axes x1y1 title '$X~(mm)=-910$' w yerrorbars lc rgb '#FF0000'  pt 1 ps 1.0  lw 1.0  lt 1 ,\\\nfile index 0 using 1:2:3 axes x1y1 title '' w lines lc rgb '#FF0000'  pt 1 ps 1.0  lw 1.0  lt 1 ,\\\nfile index 1 using 1:2:3 axes x1y1 title '$X~(mm)=-630$' w yerrorbars lc rgb '#0041DC'  pt 2 ps 1.0  lw 1.0  lt 1 ,\\\nfile index 2 using 1:2:3 axes x1y1 title '$X~(mm)=-490$' w yerrorbars lc rgb '#00C81C'  pt 3 ps 1.0  lw 1.0  lt 1"
  n1 = global read "Results_plotter_Global.vi" "Value plotted Name"() -> (w11:string)
  n2 = global read "Results_plotter_Global.vi" "Multi Ordinate?"() -> (w7:bool)
  n3 = global read "Results_plotter_Global.vi" "Plot Summary"() -> (w14:string[][])
  n4 = global read "Results_plotter_Global.vi" "Error Bar Cluster"() -> (w2:T18[])
  n5 = global read "Results_plotter_Global.vi" "X Axis Name"() -> (w13:string)
  n6 = global read "Results_plotter_Global.vi" "Y Axis Name"() -> (w12:string)
  n7 = global read "Results_plotter_Global.vi" "Transpose"() -> (w8:bool)
  n8 = while {
    shift-left: "Get Plot Folder" -> [w36]
    shift-right: [w20] -> _
    tunnel: w14 -> [w35]
    shift-right: [w34] -> _
    shift-left: _ -> [w33]
    tunnel: w13 -> [w32]
    tunnel: w12 -> [w31]
    tunnel: w11 -> [w30]
    shift-right: [w28] -> _
    shift-left: "PlotArray" -> [w29]
    shift-right: [w21] -> _
    shift-left: _ -> [w27]
    shift-right: [w26] -> _
    shift-left: _ -> [w25]
    tunnel: "terminal.log" -> [w24]
    tunnel: w8 -> [w23]
    tunnel: w7 -> [w22]
    tunnel: [w20] -> w6 mode=indexing
    tunnel: "PlotType" -> [w19]
    tunnel: "Legend Options" -> [w18]
    tunnel: w2 -> [w17]
    tunnel: "Error Bar Type" -> [w16]
    stop <- w37 continue-if-true
    n9 = case shown="\"Sort out page title\"" w36 {
      selector: w36 -> [w38 _ _ _ _ _ _ _ _ _ _ _ _ _ _ _ _ _ _ _ _]
      tunnel: [FALSE TRUE TRUE ("Top Level") TRUE ("Top Level") TRUE ("Top Level") TRUE ("Top Level") TRUE TRUE TRUE ("Top Level") TRUE ("Top Level") TRUE ("Top Level") TRUE ("Top Level") TRUE ("Top Level") TRUE ("Top Level") TRUE ("Top Level") TRUE ("Top Level") TRUE ("Top Level") TRUE ("Top Level") FALSE ("Top Level") TRUE ("Top Level") FALSE ("Top Level")] -> w37
      tunnel: ["Initialise" "FirstGuessPath" "Sort out page title" w111 w147 "Create plot directory" w162 "Save .dat file" "Save .dat file" "MakePlotTitles" "Gnuplot script Start" w332 "Build Plot Commands" "Build Plot Commands" "Write gnuplot file" ("t") "Execute shell script" ("t") "Has pdf been generated?" ("t") w598 "End" "End" ("t") "End" ("t")] -> w20
      tunnel: w35 -> [_ _ _ w106 _ _ _ _ _ w226 _ _ _ _ _ _ _ _ _ _ _]
      tunnel: [w42 w57 w96 w113 w148 w154 w167 w187 w212 w227 w249 w323 w348 w374 w429 w577 w585 w593 w606 w616 w627] -> w34
      tunnel: w33 -> [w42 _ w92 w112 w144 w155 w166 w187 w212 w227 w249 w323 w348 w374 w429 w577 w585 w593 w606 w616 w627]
      tunnel: w32 -> [_ _ _ _ _ _ _ _ _ w225 w243 _ _ _ _ _ _ _ _ _ _]
      tunnel: w31 -> [_ _ _ _ _ _ _ _ _ w224 w242 _ _ _ _ _ _ _ _ _ _]
      tunnel: w30 -> [_ _ _ _ _ _ _ _ _ _ _ _ _ _ _ _ _ _ _ _ _]
      tunnel: w29 -> [w41 w53 w95 w119 w146 w158 w170 w182 w208 w221 w248 w335 w347 w375 w387 w583 w590 w604 w611 w621 w626]
      tunnel: [w41 w53 w95 w119 w146 w158 w170 w181 w207 w221 w248 w335 w347 w375 w387 w583 w590 w604 w611 w621 w626] -> w28
      tunnel: w27 -> [w40 w56 w94 w117 w145 w157 w169 w186 w213 w228 w247 _ w341 w369 w421 w573 w588 w602 w609 w619 w625]
      tunnel: [w40 w56 w94 w117 w145 w157 w169 w186 w213 w228 w247 w309 w343 w370 w427 w573 w588 w602 w609 w619 w625] -> w21
      tunnel: [w39 w52 w93 w118 w143 w156 w168 w185 w211 w223 w246 w334 w346 w373 w428 w578 w589 w603 w610 w620 w624] -> w26
      tunnel: w25 -> [w39 _ w93 w118 w143 w156 w168 w185 w211 w223 w246 w334 w346 w373 w428 w578 w589 w603 w610 w620 w624]
      tunnel: w24 -> [_ _ _ _ _ _ _ _ _ _ _ _ _ _ _ _ w584 _ _ w614 _]
      tunnel: w23 -> [_ _ _ _ _ _ _ _ _ w222 _ _ _ _ w394 _ _ _ _ _ _]
      tunnel: w22 -> [_ _ _ _ _ _ _ _ _ _ _ _ _ _ _ _ _ _ _ _ _]
      tunnel: w19 -> [_ _ _ _ _ _ w163 _ _ _ _ w310 _ _ w386 _ _ _ _ _ _]
      tunnel: w18 -> [_ _ _ _ _ _ _ _ _ _ _ w312 _ _ w397 _ _ _ _ _ _]
      tunnel: w17 -> [_ _ _ _ _ _ _ _ _ w218 _ _ _ _ w395 _ _ _ _ _ _]
      tunnel: w16 -> [_ _ _ _ _ _ _ _ _ w217 _ _ _ _ w385 _ _ _ _ _ _]
      frame "No Match", Default {
        n10 = Current VI's Path() -> (path=w44:path)
        n11 = Format Into String(format string="The Case\"%s\" was not Matched\nin VI named\n'%s\"" ("Format String"), w38, w44) -> (resulting string=w47:string)  [unwired: 2 in, 1 out]
        n12 = One Button Dialog(message=w47, button name ("OK")="STOP") -> (true=w45:bool)
        n13 = Stop(stop? (T)=w45) -> ()
      }
      frame "Get Plot Folder" {
        n14 = case shown="True" "Set bounds using XY Plot \non Results file plotter" {
          frame False {
          }
          frame True {
            w62 = T14 {"Auto"=FALSE, "Value"=0.0} ("Min")
            n15 = local read "yAxisBounds"() -> (w61:T13)
            n16 = local read "xAxisBounds"() -> (w72:T13)
            n17 = global read "Results_plotter_Global.vi" "X plot min"() -> (w67:dbl)
            n18 = global read "Results_plotter_Global.vi" "X plot max"() -> (w68:dbl)
            n19 = global read "Results_plotter_Global.vi" "Y plot min"() -> (w66:dbl)
            n20 = global read "Results_plotter_Global.vi" "Y plot max"() -> (w65:dbl)
            n21 = Bundle By Name(cluster=w62, "Value"=w68) -> (w70:T14)
            n22 = Bundle By Name(cluster=w62, "Value"=w67) -> (w71:T14)
            n23 = Bundle By Name(cluster=w62, "Value"=w65) -> (w64:T14)
            n24 = Bundle By Name(cluster=w62, "Value"=w66) -> (w63:T14)
            n25 = Bundle By Name(cluster=w72, "Min"=w71, "Max"=w70) -> (w69:T13)
            n26 = Bundle By Name(cluster=w61, "Min"=w63, "Max"=w64) -> (w60:T13)
            n27 = local write "yAxisBounds"(w60) -> ()
            n28 = local write "xAxisBounds"(w69) -> ()
          }
        }
        n29 = global read "Results_plotter_Global.vi" "Legend"() -> (w52:string[])
        n30 = Build Path(base path="Job Directory", name or relative path="gnuplots") -> (appended path=w57:path)
        n31 = Array Size(array=w52) -> (size(s)=→"No of Series supplied":i32)
      }
      frame "FirstGuessPath" {
        w73 = ""
        n32 = global read "Results_plotter_Global.vi" "Current Data Filenames"() -> (w82:string)
        n33 = call "Fast_string_Replace.vi"("Replace match with:"="_", "Input String"=w82, "regular expression"="[/]") -> ("Output String"=w85:string)  [unwired: 2 out]
        n34 = call "Fast_string_Replace.vi"("Replace match with:"="_", "Input String"=w85, "regular expression"="__") -> ("Output String"=w83:string)  [unwired: 2 out]
        n35 = call "Fast_string_Replace.vi"("Replace match with:"=w73, "Input String"=w83, "regular expression"=" ") -> ("Output String"=w78:string)  [unwired: 2 out]
        n36 = call "Fast_string_Replace.vi"("Replace match with:"=w73, "Input String"=w78, "regular expression"="[.]") -> ("Output String"=w75:string)  [unwired: 2 out]
        n37 = call "Fast_string_Replace.vi"("Replace match with:"=w73, "Input String"=w75, "regular expression"=";") -> ("Output String"=w74:string)  [unwired: 2 out]
        n38 = String Subset(string=w74, offset (0)=0, length (rest)=30 ("length (rest)")) -> (substring=w77:string)
        n39 = Build Path(base path=w92, name or relative path=w77) -> (appended path=w96:path)
      }
      frame "Sort out page title" {
        n40 = call "DistillTitle.vi"("Plot Summary in"=w106, "Show Channels with range of Values?"="Show Channels with range of Values?", "Indices to include in Page Title"="Values to include in Page Title", "String in"="") -> ("String out"=w110:string, "AvailableVariables"=w104:string[])  [unwired: 6 in]
        n41 = property on="Values to include in Page Title" class="LstBox (strict)"("Item Names"=w104) -> ()  [unwired: 2 in, 2 out]
        n42 = Concatenate Strings("Page Title Pre Block", w110, "Page Title Post Block") -> (w100:string)
        n43 = call "Fast_string_Replace.vi"("Replace match with:"=" and " ("Individual Characters to Remove"), "Input String"=w100, "regular expression"="&" ("Individual Characters to Remove")) -> ("Output String"=w97:string)  [unwired: 1 in, 1 out]
        n44 = Current VI's Path() -> (path=w116:path)
        n45 = call "Running_as_top_level.vi"("Vi path name"=w116) -> ("Top Level"=w114:bool)  [unwired: 1 out]
        n46 = call "Any_Char_Remove.vi"("Individual Characters to Remove"="{}^&", "String in"=w97) -> ("String out"=→"Final Title":string)  [unwired: 1 in]
        n47 = case shown="True" w114 {
          tunnel: [w121 w124] -> w113
          tunnel: w112 -> [w121 _]
          tunnel: ["Get Filename" ("t") "Create plot directory"] -> w111
          frame False {
          }
          frame True {
            n48 = local read "File Path Control"() -> (w123:path)
            n49 = Strip Path(path=w123) -> (name=w122:string)  [unwired: 1 out]
            n50 = Build Path(base path=w123, name or relative path=w122) -> (appended path=w124:path)
          }
        }
      }
      frame "Get Filename" {
        n51 = local read "Final Title"() -> (w133:string)
        n52 = call "Fast_string_Replace.vi"("Replace match with:"="", "Input String"=w133, "regular expression"="~") -> ("Output String"=w130:string)  [unwired: 1 in, 1 out]
        n53 = String Length(string=w130) -> (length=w135:i32)
        n54 = case shown="1, Default" w135 {
          tunnel: [w150 w151] -> w134
          tunnel: w130 -> [w150 w153]
          frame 0 {
          }
          frame 1, Default {
            n55 = Concatenate Strings(w153, "_") -> (w151:string)
          }
        }
        n56 = call "Auto_filename.vi"("Filename Max length"="Filename Max length", "Prefix"=w134) -> ("Filename"=w137:string)
        n57 = call <vilib>:"Is Name Multiplatform.vi"("filename must be valid on all platforms (F)"=TRUE ("name must work for all platforms (F)"), "filename"=w137) -> ("filename not crossplatform"=→"crossplatform problem":bool, "filename had conflict"=→"original name had conflict":bool, "suggested filename"=w129:string)  [unwired: 5 in, 2 out]
        n58 = Build Path(base path=w144, name or relative path=w129) -> (appended path=w141:path)
        n59 = Build Path(base path=w141, name or relative path=w129) -> (appended path=w148:path)
        n60 = File/Directory Info(path=w141) -> (error out=w142:errorcluster)  [unwired: 1 in, 6 out]
        n61 = Unbundle By Name(w142) -> ("status"=w140:bool)
        n62 = Select(t="Create plot directory", s=w140, f="Find a unique name") -> (s? t:f=w147:string)
      }
      frame "Find a unique name" {
        n63 = call "FindUniqueName.vi"("Max Length"=27, "PathIn"=w155) -> ("UniquedPath"=w154:path)  [unwired: 9 in]
      }
      frame "Create plot directory" {
        n64 = call "Create_directory_path.vi"("Path name"=w166) -> ("Path name Out"=w167:path)  [unwired: 2 in, 1 out]
        n65 = Strip Path(path=w166) -> (stripped path=→"File Path Control":path)  [unwired: 1 out]
        n66 = case shown="\"XY\", Default" w163 {
          tunnel: ["Sort plot points" "AddWrapforPolar"] -> w162
          frame "XY", Default {
          }
          frame "Polar" {
          }
        }
      }
      frame "Sort plot points" {
        # "Gnuplot   uses 1/1/1970 as its datum time rather than the labview value of 1/1/1904 which is 2082844800 seconds different"
        n67 = call "TimeWizard_NoSearch.vi"("Time/Date Format"="Time/Date Format", "Select Time Zone"="Select Time Zone") -> ("Format String"=→"Time Format String":string, "Formatted date/time string"=→"Formatted date/time string":string, "TZ Shift (hrs)"=→"TZ Shift (hrs)":string, "TZ Shift (sec)"=w173:dbl)  [unwired: 1 in]
        n68 = for {
          tunnel: w182 -> [w196] mode=indexing
          tunnel: [w197] -> w181 mode=indexing
          tunnel: [w189] -> w184 mode=indexing
          tunnel: w173 -> [w188]
          n69 = Unbundle(w196) -> ("Angle"=w192:dbl[], "Radius"=w193:dbl[])
          n70 = Array Max & Min(array=w192) -> (max value=w195:dbl)  [unwired: 3 out]
          n71 = Greater?(x=w195, y=2680560000.0) -> (0:w190:bool)
          n72 = case shown="True" w190 {
            tunnel: w192 -> [w199 w205]
            tunnel: [w199 w201] -> w191
            tunnel: [FALSE TRUE] -> w189
            tunnel: w188 -> [_ w200]
            frame False {
            }
            frame True {
              w204 = 2082844800.0  # datumOffset(s)
              n73 = Subtract(x=w205, y=w204) -> (x-y=w203:dbl[])
              n74 = Add(x=w203, y=w200) -> (x+y=w201:dbl[])
            }
          }
          n75 = Bundle("Angle"=w191, "Radius"=w193) -> (w197:cluster{"Angle":dbl[], "Radius":dbl[]})  [unwired: 1 out]
        }
        n76 = Or Array Elements(Boolean array=w184) -> (logical OR=→"Time format?":bool)
      }
      frame "AddWrapforPolar" {
        n77 = for {
          tunnel: w208 -> [w216] mode=indexing
          tunnel: [w215] -> w207 mode=indexing
          tunnel: "wrapGapsUpTo:" -> [w214]
          # "Wrap plot if gap <=30deg"
          n78 = call "WrapPolarPlot.vi"("maxWrap"=w214, "thetaRin"=w216) -> ("thetaRout"=w215:cluster{"Angle":dbl[], "Radius":dbl[]})  [unwired: 9 in]
        }
      }
      frame "Save .dat file" {
        n79 = call "MakeDataFileForMultiplot.vi"("Legend"=w223, "Path"=w227, "Plot Array"=w221, "Plot Summary"=w226, "Transpose"=w222, "Error Bar Cluster"=w218, "X Axis Name"=w225, "Y Axis Name"=w224, "Error Bar Type"=w217) -> ()  [unwired: 7 in]
      }
      frame "MakePlotTitles" {
        (unwired) "-uw/U_{ref}^2__Uref (m/s)=1__LDA X (mm)=0__"
        n80 = global read "Results_plotter_Global.vi" "Filter 1 Strings"() -> (w229:string[])
        n81 = global read "Results_plotter_Global.vi" "Ordinate Strings"() -> (w236:string[])
        n82 = global read "Results_plotter_Global.vi" "Filter 2 Strings"() -> (w232:string[])
        n83 = call "TypesetInsideMathmode.vi"("DirtyString"=w243) -> ("Mathmode String"=→"X or theta label":string)  [unwired: 8 in, 2 out]
        n84 = call "TypesetInsideMathmode.vi"("DirtyString"=w242) -> ("Mathmode String"=→"Y or R label":string)  [unwired: 8 in, 2 out]
        n85 = call "makeNames.vi"("Strings"=w229) -> ("Names"=w230:string[])  [unwired: 10 in]
        n86 = Array Size(array=w236) -> (size(s)=w235:i32)
        n87 = call "makeNames.vi"("Strings"=w232) -> ("Names"=w231:string[])  [unwired: 10 in]
        n88 = Greater?(x=w235, y=1) -> (0:w233:bool)
        "Multi_Plot" <- w233
        n89 = case shown="True" w233 {
          tunnel: w230 -> [w253 w291]
          tunnel: w231 -> [w254 w292]
          tunnel: [w250 w295] -> w239
          tunnel: [w257 w294] -> w238
          tunnel: [w258 w293] -> w237
          tunnel: w236 -> [w257 _]
          frame True {
            n90 = Array Size(array=w253) -> (size(s)=w256:i32)
            n91 = Array Size(array=w254) -> (size(s)=w255:i32)
            n92 = Greater?(x=w256, y=w255) -> (0:w252:bool)
            n93 = case shown="False" w252 {
              tunnel: [w266 w281] -> w258
              tunnel: w257 -> [w265 w280]
              tunnel: w254 -> [w263 w279]
              tunnel: w253 -> [w264 w277]
              tunnel: [w263 w277] -> w251
              frame False {
                n94 = Index Array(array=w264) -> (element=w267:string)  [unwired: 1 in]
                n95 = for {
                  tunnel: w267 -> [w271]
                  tunnel: w263 -> [w270]
                  tunnel: [w269] -> w266 mode=indexing
                  tunnel: w265 -> [w268] mode=indexing
                  n96 = for {
                    tunnel: w271 -> [w276]
                    tunnel: w270 -> [w275] mode=indexing
                    tunnel: [w274] -> w269 mode=indexing
                    tunnel: w268 -> [w273]
                    w272 = "__" ("string")
                    n97 = Concatenate Strings(w273, w272, w276, w272, w275, w272) -> (w274:string)
                  }
                }
              }
              frame True {
                n98 = Index Array(array=w279) -> (element=w278:string)  [unwired: 1 in]
                n99 = for {
                  tunnel: w277 -> [w285]
                  tunnel: w278 -> [w284]
                  tunnel: [w283] -> w281 mode=indexing
                  tunnel: w280 -> [w282] mode=indexing
                  n100 = for {
                    tunnel: w285 -> [w290] mode=indexing
                    tunnel: w284 -> [w289]
                    tunnel: [w288] -> w283 mode=indexing
                    tunnel: w282 -> [w287]
                    w286 = "__" ("string")
                    n101 = Concatenate Strings(w287, w286, w290, w286, w289, w286) -> (w288:string)
                  }
                }
              }
            }
            n102 = for {
              tunnel: w251 -> [w261] mode=indexing
              tunnel: [w260] -> w250 mode=indexing
              n103 = call "Fast_string_Replace.vi"("Replace match with:"="~", "Input String"=w261, "regular expression"="_") -> ("Output String"=w260:string)  [unwired: 1 in, 1 out]
            }
          }
          frame False {
            n104 = for {
              tunnel: w291 -> [w304]
              tunnel: w292 -> [w303] mode=indexing
              tunnel: [w302] -> w293 mode=indexing
              n105 = for {
                tunnel: w304 -> [w308] mode=indexing
                tunnel: w303 -> [w307]
                tunnel: [w305] -> w302 mode=indexing
                w306 = "__" ("string")
                n106 = Concatenate Strings(w308, w306, w307, w306) -> (w305:string)
              }
            }
            n107 = for {
              tunnel: w292 -> [w301] mode=indexing
              tunnel: [w300] -> w294 mode=indexing
              # "Put space back in either side of the = sign"
              n108 = call "Edit_First_Equal.vi"("String in"=w301) -> ("String out"=w300:string)
            }
            n109 = for {
              tunnel: w291 -> [w297] mode=indexing
              tunnel: [w296] -> w295 mode=indexing
              n110 = call "Fast_string_Replace.vi"("Replace match with:"=" ", "Input String"=w297, "regular expression"="_") -> ("Output String"=w296:string)  [unwired: 2 out]
            }
          }
        }
        "AutoPlotTitles" <- w238
        "Plot Legends Auto" <- w239
        "Desired Legends" <- w237
      }
      frame "Gnuplot script Start" {
        n111 = local read "GraphPeripherals"() -> (w317:T17[][])
        n112 = call "setTerm.vi"("Height (in)"="Height (in)", "Width (in)"="Width (in)", "String in"="") -> ("String out"=w328:string)  [unwired: 7 in, 1 out]
        n113 = local read "Final Title"() -> (w326:string)
        n114 = call "setMultiplot.vi"("ScaleAdjust"="ScaleAdjust", "OverallTitle"=w326, "Cols"="nCols", "Rows"="nRows", "String in"=w328) -> ("nGraphs"=→"No of Graph Slots Available":i32, "String out"=w327:string)  [unwired: 4 in, 1 out]
        n115 = call "perpheralsInitialise.vi"("Legend"=w312, "PeripheralsMasterControl"="PeripheralsMasterControl", "Cols"="nCols", "Rows"="nRows", "GraphPeripheralsIn"=w317) -> ("GraphPeripheralsOut"=w318:T17[][])  [unwired: 6 in]
        n116 = local write "GraphPeripherals"(w318) -> ()
        n117 = call "setMargins.vi"("Margins"="Margins", "String in"=w327) -> ("String out"=w314:string)  [unwired: 8 in, 1 out]
        n118 = call "chainCommands.vi"("Command"="set style line 12 lc rgb '#C0C0C0' lt 1 lw 1.5 # useful pale linestyle for grids", "StringIn"=w314) -> ("StringOut"=w315:string)  [unwired: 9 in]
        n119 = Strip Path(path=w323) -> (name=w322:string)  [unwired: 1 out]
        n120 = Format Into String(format string="file=\"%s.dat\"\n" ("string"), initial string=w315, w322) -> (resulting string=w309:string)  [unwired: 1 in, 1 out]
        n121 = case shown="\"XY\", Default" w310 {
          tunnel: ["XYPlot" "PolarPlot"] -> w332
          frame "XY", Default {
          }
          frame "Polar" {
          }
        }
      }
      frame "XYPlot" {
        n122 = case shown="\"True\"" "Additional XYgnuplot" {
          selector: "Additional XYgnuplot" -> [w349 w353]
          tunnel: [w349 w352] -> w339
          frame "", Default {
          }
          frame "True" {
            n123 = Concatenate Strings("# Manual gnuplot Start" ("string"), w353, "# Manual gnuplot End" ("string")) -> (w352:string)
          }
        }
        n124 = Concatenate Strings(w341, "set border ls 12\n" ("input 2"), w339) -> (w343:string)
        "PlotCommand" <- "file index %d using 1:2 axes x1y1 title '%s' w " ("format string")
      }
      frame "PolarPlot" {
        n125 = case shown="\"True\"" "Additional Polar gnuplot" {
          selector: "Additional Polar gnuplot" -> [w378 w382]
          tunnel: [w378 w381] -> w358
          frame "", Default {
          }
          frame "True" {
            n126 = Concatenate Strings("# Manual gnuplot Start" ("string"), w382, "# Manual gnuplot End" ("string")) -> (w381:string)
          }
        }
        n127 = Select(t="set angles degrees\n", s="Angle Units", f="set angles radians\n") -> (s? t:f=w360:string)
        n128 = case shown="\"Compass\"" "AngleMode" {
          tunnel: ["90-$1" ("format string") "$1" ("format string")] -> w365
          frame "Compass" {
          }
          frame "Math", Default {
          }
        }
        n129 = Concatenate Strings(w369, w360, "set polar\nset size square\n", w358) -> (w370:string)
        n130 = case shown="\"Compass\"" "AngleMode" {
          tunnel: [90.0 0.0] -> w355
          frame "Compass" {
          }
          frame "Math", Default {
          }
        }
        n131 = Concatenate Strings("file index %d using (" ("format string"), w365, "):2 axes x1y1 title '%s' w " ("format string")) -> (w364:string)
        n132 = local read "X/Theta tics And Grids"() -> (w357:T10)
        n133 = Bundle By Name(cluster=w357, "tics.ticMin"=w355) -> (w356:T10)
        n134 = local write "PlotCommand"(w364) -> ()
        n135 = local write "X/Theta tics And Grids"(w356) -> ()
      }
      frame "Build Plot Commands" {
        n136 = local read "Desired Legends"() -> (w393:string[][])
        n137 = local read "Plot Legends Auto"() -> (w399:string[])
        n138 = Array Size(array=w393) -> (size(s)=w392:i32[])
        n139 = Index Array(array=w392) -> (element=w391:i32)  [unwired: 1 in]
        n140 = local read "AutoPlotTitles"() -> (w419:string[])
        n141 = case shown="\"Autolabel\", Default" "Y axis label" {
          tunnel: [w430 "Y or R label Manual 2"] -> w404
          frame "Autolabel", Default {
            n142 = local read "Y or R label"() -> (w430:string)
          }
          frame "Manual Label" {
          }
        }
        n143 = case shown="\"Autolabel\", Default" "X axis label" {
          tunnel: [w439 "X or theta label Manual"] -> w409
          frame "Autolabel", Default {
            n144 = local read "X or theta label"() -> (w439:string)
          }
          frame "Manual Label" {
          }
        }
        n145 = Select(t=w399, s="Plot Legends", f="Plot Legends Manual") -> (s? t:f=w398:string[])
        n146 = case shown="Default" w386 {
          tunnel: [T19 "theta" ("Axis") T19 "x" ("Axis")] -> w407
          tunnel: [T19 "r" ("Axis") T19 "y" ("Axis")] -> w406
          tunnel: ["rAxisBounds" "yAxisBounds"] -> w408
          tunnel: ["rAxisBounds" "xAxisBounds"] -> w388
          frame "Polar" {
          }
          frame Default {
          }
        }
        n147 = local read "PlotCommand"() -> (w411:string)
        n148 = global read "Results_plotter_Global.vi" "Legend"() -> (w415:string[])
        n149 = call "serialiseArray.vi"("GraphPeripherals"="GraphPeripherals") -> ("output array"=w416:T17[])  [unwired: 10 in]
        n150 = Select(t=w419, s="Individual Plot Titles", f="ManualPlotTitles") -> (s? t:f=w396:string[])
        n151 = for {
          shift-right: [w448] -> w422
          shift-left: "\n#Begin plots\n" -> [w473]
          tunnel: w398 -> [w474]
          tunnel: "Plotstyles" -> [w475]
          tunnel: w396 -> [w471] mode=indexing
          tunnel: w416 -> [w472] mode=indexing
          tunnel: w393 -> [w444] mode=indexing
          tunnel: w415 -> [w442]
          tunnel: "LegendProperties" -> [w461]
          tunnel: "Plot Title Offset (characters)" -> [w470]
          tunnel: w411 -> [w469]
          tunnel: w409 -> [w468]
          tunnel: w408 -> [w467]
          tunnel: w407 -> [w466]
          tunnel: w406 -> [w465]
          tunnel: w404 -> [w464]
          tunnel: "Y/R tics And Grids" -> [w463]
          tunnel: "X/Theta tics And Grids" -> [w462]
          tunnel: w387 -> [w446]
          tunnel: w397 -> [w460]
          tunnel: w395 -> [w456]
          tunnel: w394 -> [w455]
          tunnel: w391 -> [w454]
          tunnel: "PlotNamesNeed $$?" -> [w453]
          tunnel: "PlotTitlesNeed $$?" -> [w452]
          tunnel: w388 -> [w451]
          tunnel: w386 -> [w447]
          tunnel: w387 -> [w445]
          tunnel: w386 -> [w443]
          tunnel: w385 -> [w441]
          i -> [w459]
          # "Loops once for each graph on the multiplot"
          n152 = call "BuildPlotsOneGraph.vi"("PlotCommand"=w469, "Desired Legends"=w444, "Error Bar Type"=w441, "Plotstyles"=w475, "PlotNamesNeed $$?"=w453, "Plot Legends"=w474, "PlotArray"=w446, "Legend"=w442, "Error Bar Cluster"=w456) -> ("String out"=w449:string, "Xspan"=w457:cluster{"Max":dbl, "Min":dbl}, "Yspan"=w458:cluster{"Max":dbl, "Min":dbl})  [unwired: 4 in]
          n153 = stacked-sequence {
            seq-local: [w486 _] -> [_ w542]
            seq-local: [w482 _] -> [_ w541]
            tunnel: [_ w556] -> w450
            tunnel: w449 -> [_ w520]
            tunnel: w473 -> [_ w555]
            tunnel: w472 -> [w484 w554]
            tunnel: w471 -> [_ w547]
            tunnel: w470 -> [_ w546]
            tunnel: w468 -> [_ w533]
            tunnel: w467 -> [_ w540]
            tunnel: w466 -> [_ w545]
            tunnel: w465 -> [_ w544]
            tunnel: w464 -> [_ w537]
            tunnel: w463 -> [_ w543]
            tunnel: w462 -> [_ w526]
            tunnel: w461 -> [w485 _]
            tunnel: w460 -> [w487 _]
            tunnel: w459 -> [w481 _]
            tunnel: w458 -> [_ w538]
            tunnel: w457 -> [_ w539]
            tunnel: w455 -> [_ w532]
            tunnel: w454 -> [w480 _]
            tunnel: w452 -> [_ w530]
            tunnel: w451 -> [_ w527]
            tunnel: w445 -> [_ _]
            tunnel: w443 -> [_ w521]
            frame #0 {
              n154 = Unbundle By Name(w484) -> ("key"=w483:bool)
              n155 = case shown="\"Single Legend Below table\"" w487 {
                tunnel: [w489 w493] -> w486
                tunnel: w485 -> [w489 w494]
                tunnel: w483 -> [w488 _]
                tunnel: [w488 w492] -> w482
                tunnel: w481 -> [_ w490]
                tunnel: w480 -> [_ w491]
                frame "Legend as per array", Default {
                }
                frame "Single Legend Below table" {
                  n156 = stacked-sequence {
                    seq-local: [w496 _] -> [_ w513]
                    seq-local: [w495 _] -> [_ w512]
                    tunnel: w494 -> [_ w519]
                    tunnel: w490 -> [_ w516]
                    tunnel: [_ w515] -> w493
                    tunnel: [_ w514] -> w492
                    tunnel: w491 -> [w498 _]
                    frame #0 {
                      n157 = local read "No of Graph Slots Available"() -> (w499:i32)
                      n158 = Greater?(x=w499, y=w498) -> (0:w497:bool)
                      n159 = case shown="True" w497 {
                        tunnel: [0.6 ("\"At\" location.Xvalue") w506] -> w496
                        tunnel: [-0.03 ("\"At\" location.Yvalue") w503] -> w495
                        frame False {
                        }
                        frame True {
                          n160 = local read "nCols"() -> (w510:u8)
                          n161 = local read "nRows"() -> (w504:u8)
                          n162 = Decrement(x=w510) -> (x-1=w511:u8)
                          n163 = Increment(x=w504) -> (x+1=w502:u8)
                          n164 = Divide(x=w511, y=w510) -> (x/y=w507:dbl)
                          n165 = Divide(x=1.0, y=w502) -> (x/y=w503:dbl)
                          n166 = Divide(x=0.7, y=w510) -> (x/y=w508:dbl)
                          n167 = Add(x=w507, y=w508) -> (x+y=w506:dbl)
                        }
                      }
                    }
                    frame #1 {
                      w517 = "screen" ("\"At\" location.XcoordSys")
                      # "Use \"screen\" coordinates to place legend at bottom-center\nof entire \"screen\" of graphs; update legend cluster to \nreflect this."
                      # "Only legend the first graph"
                      n168 = Equal To 0?(x=w516) -> (x = 0?=w514:bool)
                      n169 = Bundle By Name(cluster=w519, "Location"="at", "\"At\" location.XcoordSys"=w517, "\"At\" location.Xvalue"=w513, "\"At\" location.YcoordSys"=w517, "\"At\" location.Yvalue"=w512) -> (w515:T6)
                      n170 = local write "LegendProperties"(w515) -> ()
                    }
                  }
                }
              }
            }
            frame #1 {
              n171 = local read "Multi_Plot"() -> (w535:bool)
              n172 = case shown="False" w532 {
                tunnel: w537 -> [w563 w572]
                tunnel: [w563 w571] -> w536
                tunnel: w535 -> [w566 w569]
                tunnel: [w564 w568] -> w534
                tunnel: w533 -> [w565 w568]
                frame True {
                  n173 = Select(t="", s=w566, f=w565) -> (s? t:f=w564:string)
                }
                frame False {
                  n174 = Select(t="", s=w569, f=w572) -> (s? t:f=w571:string)
                }
              }
              n175 = Unbundle By Name(w554) -> ("title"=w553:bool, "Xtic"=w551:bool, "Xlab"=w550:bool, "Ytic"=w549:bool, "Ylab"=w548:bool)
              n176 = call "TypesetInsideMathmode.vi"("Needs $$?"=w530, "DirtyString"=w547) -> ("ChosenStringtype"=w531:string)  [unwired: 7 in, 2 out]
              n177 = call "setTitle.vi"("Offset"=w546, "Set?"=w553, "Title"=w531, "String in"=w555) -> ("String out"=w552:string)  [unwired: 6 in, 1 out]
              n178 = local read "Time Format String"() -> (w528:string)
              n179 = local read "Time format?"() -> (w529:bool)
              n180 = call "setKey.vi"("LegendProperties"=w542, "Set?"=w541, "String in"=w552) -> ("String out"=w525:string)  [unwired: 7 in, 1 out]
              n181 = call "AxisControl.vi"("String in"=w525, "AxisBounds"=w540, "ticsAndGrids"=w543, "Axis"=w544, "ShowNumbers?"=w549, "ShowLabel?"=w548, "Axis Label"=w536, "DataSpan"=w538) -> ("String out"=w523:string)  [unwired: 6 in, 1 out]
              n182 = case shown="\"Polar\"" w521 {
                tunnel: w523 -> [w557 w559]
                tunnel: [w557 w558] -> w522
                tunnel: w520 -> [_ w560]
                frame "XY", Default {
                }
                frame "Polar" {
                  n183 = Concatenate Strings(w559, "set table \"outfile.txt\"\n" ("string"), w560, "rmax = GPVAL_R_MAX\nrmin = GPVAL_R_MIN\nunset table\n" ("string")) -> (w558:string)
                }
              }
              n184 = call "AxisControl.vi"("String in"=w522, "AxisBounds"=w527, "Time Format String"=w528, "ticsAndGrids"=w526, "Axis"=w545, "Time format?"=w529, "ShowNumbers?"=w551, "ShowLabel?"=w550, "Axis Label"=w534, "DataSpan"=w539) -> ("String out"=w524:string)  [unwired: 4 in, 1 out]
              n185 = Concatenate Strings(w524, w520) -> (w556:string)
            }
          }
          n186 = case shown="\"Polar\"" w447 {
            tunnel: w450 -> [w476 w479]
            tunnel: [w476 w478] -> w448
            frame "XY", Default {
            }
            frame "Polar" {
              n187 = Concatenate Strings(w479, "unset label\n" ("string")) -> (w478:string)
            }
          }
        }
        n188 = Concatenate Strings(w421, w422, "\nunset multiplot\n") -> (w427:string)
      }
      frame "Write gnuplot file" {
        w580 = FALSE  # append to file? (new file:F)
        w581 = FALSE  # advisory dialog? (display:T)
        n189 = Strip Path(path=w577) -> (stripped path=w574:path)  [unwired: 1 out]
        n190 = Build Path(base path=w574, name or relative path="gnuplot_script.txt") -> (appended path=w582:path)
        n191 = call "Write_Characters_To_File.vi"("file path (dialog if empty)"=w582, "advisory dialog? (display:T)"=w581, "character string"=w573, "append to file? (new file:F)"=w580) -> ()  [unwired: 1 in, 4 out]
      }
      frame "Execute shell script" {
        n192 = call "Run_Gnuplot_Script.vi"("logfileName"=w584, "workingDirectory"=w585) -> ()  [unwired: 1 in]
      }
      frame "Has pdf been generated?" {
        n193 = Current VI's Path() -> (path=w591:path)
        n194 = call "Running_as_top_level.vi"("Vi path name"=w591) -> ("Top Level"=w592:bool)  [unwired: 1 out]
        n195 = call "Create_copy_of_pdf in day folder.vi"("Top Level"=w592, "Path name Out"=w593) -> ()  [unwired: 1 in]
        n196 = Select(t="Open Standard output file" ("f"), s="OpenLogfile?", f="End") -> (s? t:f=w594:string)
        n197 = Select(t="Show Re-Run Gnuplot?", s="Show Script Editor?", f=w594) -> (s? t:f=w598:string)
      }
      frame "Show Re-Run Gnuplot?" {
        n198 = Strip Path(path=w606) -> (stripped path=w605:path)  [unwired: 1 out]
        n199 = call "Re_run_Gnuplot.vi"("Plot folder (dialog if empty)"=w605) -> ()  [unwired: 1 in, 3 out]
      }
      frame "Open Standard output file" {
        n200 = Strip Path(path=w616) -> (stripped path=w613:path)  [unwired: 1 out]
        n201 = Format Into String(format string="open \"%s\"", w614) -> (resulting string=w612:string)  [unwired: 2 in, 1 out]
        n202 = call <vilib>:"System Exec.vi"("working directory"=w613, "command line"=w612) -> ()  [unwired: 4 in, 6 out]
      }
      frame "End" {
      }
    }
    "gnuplotScript" <- w21
  }
  "AuditTrail" <- w6
  "Saved Automatically?" <- FALSE
